vi "WHD_VEten_.WS_BIDIR_Cal_26_01_2024.vi"() -> ()   [LabVIEW 2015]
uses:
  <vilib>/LabVIEW Targets/FPGA/cRIO/shared/nicrio_ModuleControls/nicrio_cRIO-9234_DataRatesRing2.ctl
  <vilib>/RTwatchdog.llb/Watchdog expiration actions.ctl
  <vilib>/userdefined/High Color/nirio_resource_hc.ctl
  <vilib>/Platform/TimedLoop/XDataNode/timing_clust.ctl
  <vilib>/Platform/TimedLoop/XDataNode/nitl_modes.ctl
  <vilib>/Platform/TimedLoop/XDataNode/wakeup.ctl
  <vilib>/Analysis/5stat.llb/RMS (DBL).vi
  <vilib>/FPGAPlugInAG/cRIO-9031/niLvFpga_Open_cRIO-9031.vi
  <vilib>/Utility/error.llb/Error Cluster From Error Code.vi
  <vilib>/rvi/errors/niLvFpgaAdjustHostInterfaceError.vi
  <vilib>/FPGAPlugInAG/cRIO-9031/niLvFpga_Run_cRIO-9031.vi
  <vilib>/rvi/interface/common/niFpgaWaitOnOcc.vi
  <vilib>/Utility/file.llb/Write Delimited Spreadsheet (string).vi
  <vilib>/FPGAPlugInAG/cRIO-9031/niLvFpga_Reset_cRIO-9031.vi
  <vilib>/measure/madcrms.llb/Basic Averaged DC-RMS for 1 Chan.vi
  <vilib>/measure/maspectr.llb/FFT Spectrum (Mag-Phase) for 1 Chan.vi
  <vilib>/Utility/config.llb/Write Key (Double).vi
  <vilib>/FPGAPlugInAG/cRIO-9031/niLvFpga_Close_cRIO-9031.vi
  <vilib>/rvi/interface/nirviOpenFPGA/nirviOpenFPGA.xnode
  FPGA Bitfiles/WRDArabia_FPGATarget_FPGA8a2wsBIdirec_pdg683fU6LY.lvbitx
  <vilib>/rvi/interface/nirviReadWriteControl/nirviReadWriteControl.xnode
  <vilib>/rvi/interface/nirviMethod/nirviMethod.xnode
  <vilib>/platform/TimedLoop/XDataNode/XDataNode.xnode
  <vilib>/rvi/interface/nirviCloseFPGA/nirviCloseFPGA.xnode
  <vilib>/rvi/errors/niLvFpgaMergeErrorWithErrorCode.vi
  AURA_Wheel/Json2Labv.lvlib
  AURA_Wheel/AuraWheelAPI/AuraWheel.lvlib
  NiFpgaLv.dll
  <vilib>/FPGAPlugInAG/cRIO-9031/niLvFpga_ConfigureFifo_cRIO-9031.vi
  <vilib>/FPGAPlugInAG/cRIO-9031/niLvFpga_StartFifo_cRIO-9031.vi
  <vilib>/FPGAPlugInAG/cRIO-9031/niLvFpga_ReadFifo_cRIO-9031.vi
  <vilib>/FPGAPlugInAG/cRIO-9031/niLvFpga_StopFifo_cRIO-9031.vi
  <vilib>/measure/NI_MAPro.lvlib
  <vilib>/Analysis/NI_AALPro.lvlib
  <vilib>/Analysis/NI_AALBase.lvlib
  <vilib>/Utility/config.llb/NI_LVConfig.lvlib
  <vilib>/Platform/TimedLoop/XDataNode/XDNodeRunTimeDep.lvlib
  Library/IF2_Reader/IF2_Reader.lvlib
panel:
  out "Power Status":bool
  out "Diagnostic data":sgl[](array[numeric])
  out "Last Train passes - RFIDs":T1
  out "I2":sgl[](array[numeric])
  out "I1":sgl[](array[numeric])
  out "A8":sgl[](array[numeric])
  out "A7":sgl[](array[numeric])
  out "A6":sgl[](array[numeric])
  out "A5":sgl[](array[numeric])
  out "A4":sgl[](array[numeric])
  out "A3":sgl[](array[numeric])
  out "A2":sgl[](array[numeric])
  out "A1":sgl[](array[numeric])
  out "Accelerometer 8":bool
  out "Accelerometer 7":bool
  out "Accelerometer 6":bool
  out "Accelerometer 5":bool
  out "Accelerometer 4":bool
  out "Accelerometer 3":bool
  out "Accelerometer 2":bool
  out "Accelerometer 1":bool
  out "Wheel detector 2":bool
  out "Wheel Detector 1":bool
  out "Last time checked":string
  out "RFID connection":bool
  out "Internet connection":bool
  out "Inicio diagnosis":timestamp
  out "RFID_status":path=path "c:/RFID/status.csv"
  in  "Diagnosis":bool
  out "T fuera rango":bool
  out "Frequency":dbl[](array[numeric])
  out "Value to compare":dbl[](array[numeric])
  in  "Developer password":string
  out "Waveform Graph":waveform(sgl)[](graph)
  out "min":dbl[](array[numeric])
  out "max":dbl[](array[numeric])
  out "median":dbl[](array[numeric])
  out "mean":dbl[](array[numeric])
  in  "Accelerometer":i32=1 min=1 max=8
  out "Low cutoff freq":dbl
  out "noise_range":dbl
  out "Numeric":i32
  out "Calibration parameter":dbl
  out "Accel.detected":i32
  out "Mean\nfrequency":dbl format="%0.2f"
  out "Nº meas":i32
  out "Array":i32[](array[numeric])
  out "sorted array":i32[](array[numeric])
  out "Array 3":i32[](array[numeric])
  out "max value":i32
  out "max index(es)":i32
  out "element":i32
  out "size(s) 3":i32
  out "size(s)":i32[](array[numeric])
  out "Valid\nindex":i32[](array[numeric])
  out "Acquiring time":dbl
  out "Inicio pasada 2":timestamp
  out "calibration log":path
  out "date/time string 2":string
  out "Folder":path
  in  "Developer commad":string
  out "Save calibration":bool
  out "Pattern amplitude (g)":dbl=1.02
  out "Pattern frequency (Hz)":dbl=159.2
  out "Report":string
  out "AURA wheel test":bool
  out "LOG.txt":path
  out "Report_AURA":string
  out "error FPGA":errorcluster
  out "error AURA":errorcluster
  out "error manipulacion archivos":errorcluster
  out "Response headers":string
  out "Max RMS Ruedas":dbl[][](array[numeric])
  out "TAGs LR6":string[](array[string])
  out "TAGs HEX":string[](array[string])
  out "Parar":bool
  out "result":bool
  out "TAGs":string[](array[string])
  out "Temperatura (ºC)":dbl
  out "V (m/s)":dbl
  out "Digital?":bool=TRUE
  out "Watchdog config":T2={"reset"=FALSE, "occurrence"=FALSE, "trigger protocol"=enum."active high", "trigger line"=enum."none", "disable watchdog on VI exit"=TRUE}
  out "Tiempo de adquisicion":dbl=10.0
  out "Adquirir":bool
  out "Nº Ruedas 1":i32
  out "NºRuedas 2":i32
  out "Disco Duro Disponible (bytes)":i64
  out "Buffer Overflow":bool
  out "Buffer Underflow":bool
  out "Archivo\nvalido?":bool
  out "Número de ejes detectados":i32
  out "Ejes_convoy":i32
  out "Tiempo de paso (s)":dbl
  out "created path":path
  out "Nombre de archivo":path[](array[path])
  out "LR6 IP address":string="192.168.106.94"
  out "Port LR6":u16=2001
  out "Frecuencia de muestreo (Hz)":dbl=25600.0
  out "Escaneos de la FIFO por canal":u32=5000
  out "Tiempo extra al detector de paso (s)":dbl=1.0
  out "dt RMS":dbl=256.0
  out "Frecuencia de muestreo y módulo CRIO":T3=2 items=["51.200 kS/s (NI 9234)"=1, "25.600 kS/s (NI 9234)"=2, "17.067 kS/s (NI 9234)"=3, "12.800 kS/s (NI 9234)"=4, "10.240 kS/s (NI 9234)"=5, "8.533 kS/s (NI 9234)"=6, "7.314 kS/s (NI 9234)"=7, "6.400 kS/s (NI 9234)"=8, "5.689 kS/s (NI 9234)"=9, "5.120 kS/s (NI 9234)"=10, "4.654 kS/s (NI 9234)"=11, "4.267 kS/s (NI 9234)"=12, "3.938 kS/s (NI 9234)"=13, "3.657 kS/s (NI 9234)"=14, "3.413 kS/s (NI 9234)"=15, "3.200 kS/s (NI 9234)"=16, "3.012 kS/s (NI 9234)"=17, "2.845 kS/s (NI 9234)"=18, "2.695 kS/s (NI 9234)"=19, "2.560 kS/s (NI 9234)"=20, "2.438 kS/s (NI 9234)"=21, "2.328 kS/s (NI 9234)"=22, "2.226 kS/s (NI 9234)"=23, "2.133 kS/s (NI 9234)"=24, "2.048 kS/s (NI 9234)"=25, "1.969 kS/s (NI 9234)"=26, "1.896 kS/s (NI 9234)"=27, "1.829 kS/s (NI 9234)"=28, "1.765 kS/s (NI 9234)"=29, "1.707 kS/s (NI 9234)"=30, "1.652 kS/s (NI 9234)"=31]
  out "Puerto RFID":u16=2189
  out "IP RFID":string="192.168.106.99"
  out "Offset_rueda WS 2":fxp<+/-,24,-4>=0.004999998956918716 format="%.27g"
  out "Count(mSec)":u32=2
  out "RFID NEM on?":bool
  out "RFID LR6 on?":bool
  out "Canal cero WS1?":bool
  out "Canal cero WS2":bool
  in  "Calibration":bool
  out "Direccion 0?":bool
  out "Boton Adquirir?":bool
  out "RuedaDetectada2?":bool=TRUE
  out "RuedaDetectada1?":bool=TRUE
  out "Timeout ruedas":dbl
  out "Borrar archivos\nadquisicion con error":bool
  out "Able watchdog?":bool
  out "Reset watchdog?":bool
  out "Leer config RFID NEM":bool
  out "bytes to read":i32
  out "DeviceAddress":u8
  out "timeout ms (60000)":i32
  out "Max archivos":u32=2
  out "Bytes libre despues de borrar":u32=2
  out "Bytes min libre":u32=2
  out "Nº de acelerómetros":i32
  out "Nº inductivos":i32
  out "Offset_rueda WS 1":fxp<+/-,24,-4>=0.004999998956918716 format="%.27g"
  out "TAGs_AURAwheel":string[][](array[string])
  out "Plataformas?":bool
  out "Nº Ejes":i32[](array[numeric])
  out "Nº UTs":i32
  out "it-read-LR6":i32[](array[numeric])
  out "it-LR6":i32
  out "RFID_LR6_Error":errorcluster
  out "Series_flota":string[](array[string])
  out "Tabla_flota":string[][](array[string])
  out "Puntos medios de las ventanas":dbl[][](array[numeric])
  out "configuration file path":path=path "c:/Parametros.cfg"
  out "IP synchr":string
  out "data":cluster{"status":string}
  out "confRFID":path=path "c:/RFID/TAGS.csv"
  out "TAGS leidos":path=path "c:/RFID/TAGS.csv"
  out "Use Aura?":bool
  out "Parametros AuraWheel":string[](array[string])
  out "Parámetros acelerómetros":dbl[](array[numeric])
  out "Fin":bool
  out "Contador":i32=1
  out "Path LOG":path=path "c:/TEST"
  out "Fallo fotocelula":bool
  out "Path_Borrar":path=path "c:/Trenes"
  out "Longitud de la unidad":dbl
  out "Aviso no detección":string
  out "Time to Acquire Block (ms)":i32
  out "Distancia de acelerómetros":dbl[](array[numeric])
  out "Block Size":u32
  out "Distancias generales":dbl[](array[numeric])
  out "Reset del controlador":bool
  out "Parar la aplicación":bool
  out "date/time string":string
  out "Timeout ruedas":bool
  out "Tiempo":dbl
  out "Inicio pasada":timestamp
  out "Ultimo TEST":timestamp
  out "DC OK":string
  out "Aviso temperatura":string
  out "connection ID":refnum<k5>
  # "To check the status of the UPS please check the following LEDs physically in the system:"
  # "10. Bar graph showing the current available supply of the UPS (each bar is a 20%)"
  # "12. Red LED: alarm"
  # "13. Yellow LED: battery working mode"
  # "16. Green LED: Power In OK, mains mode"
  # "Calibration - Noise analysis"
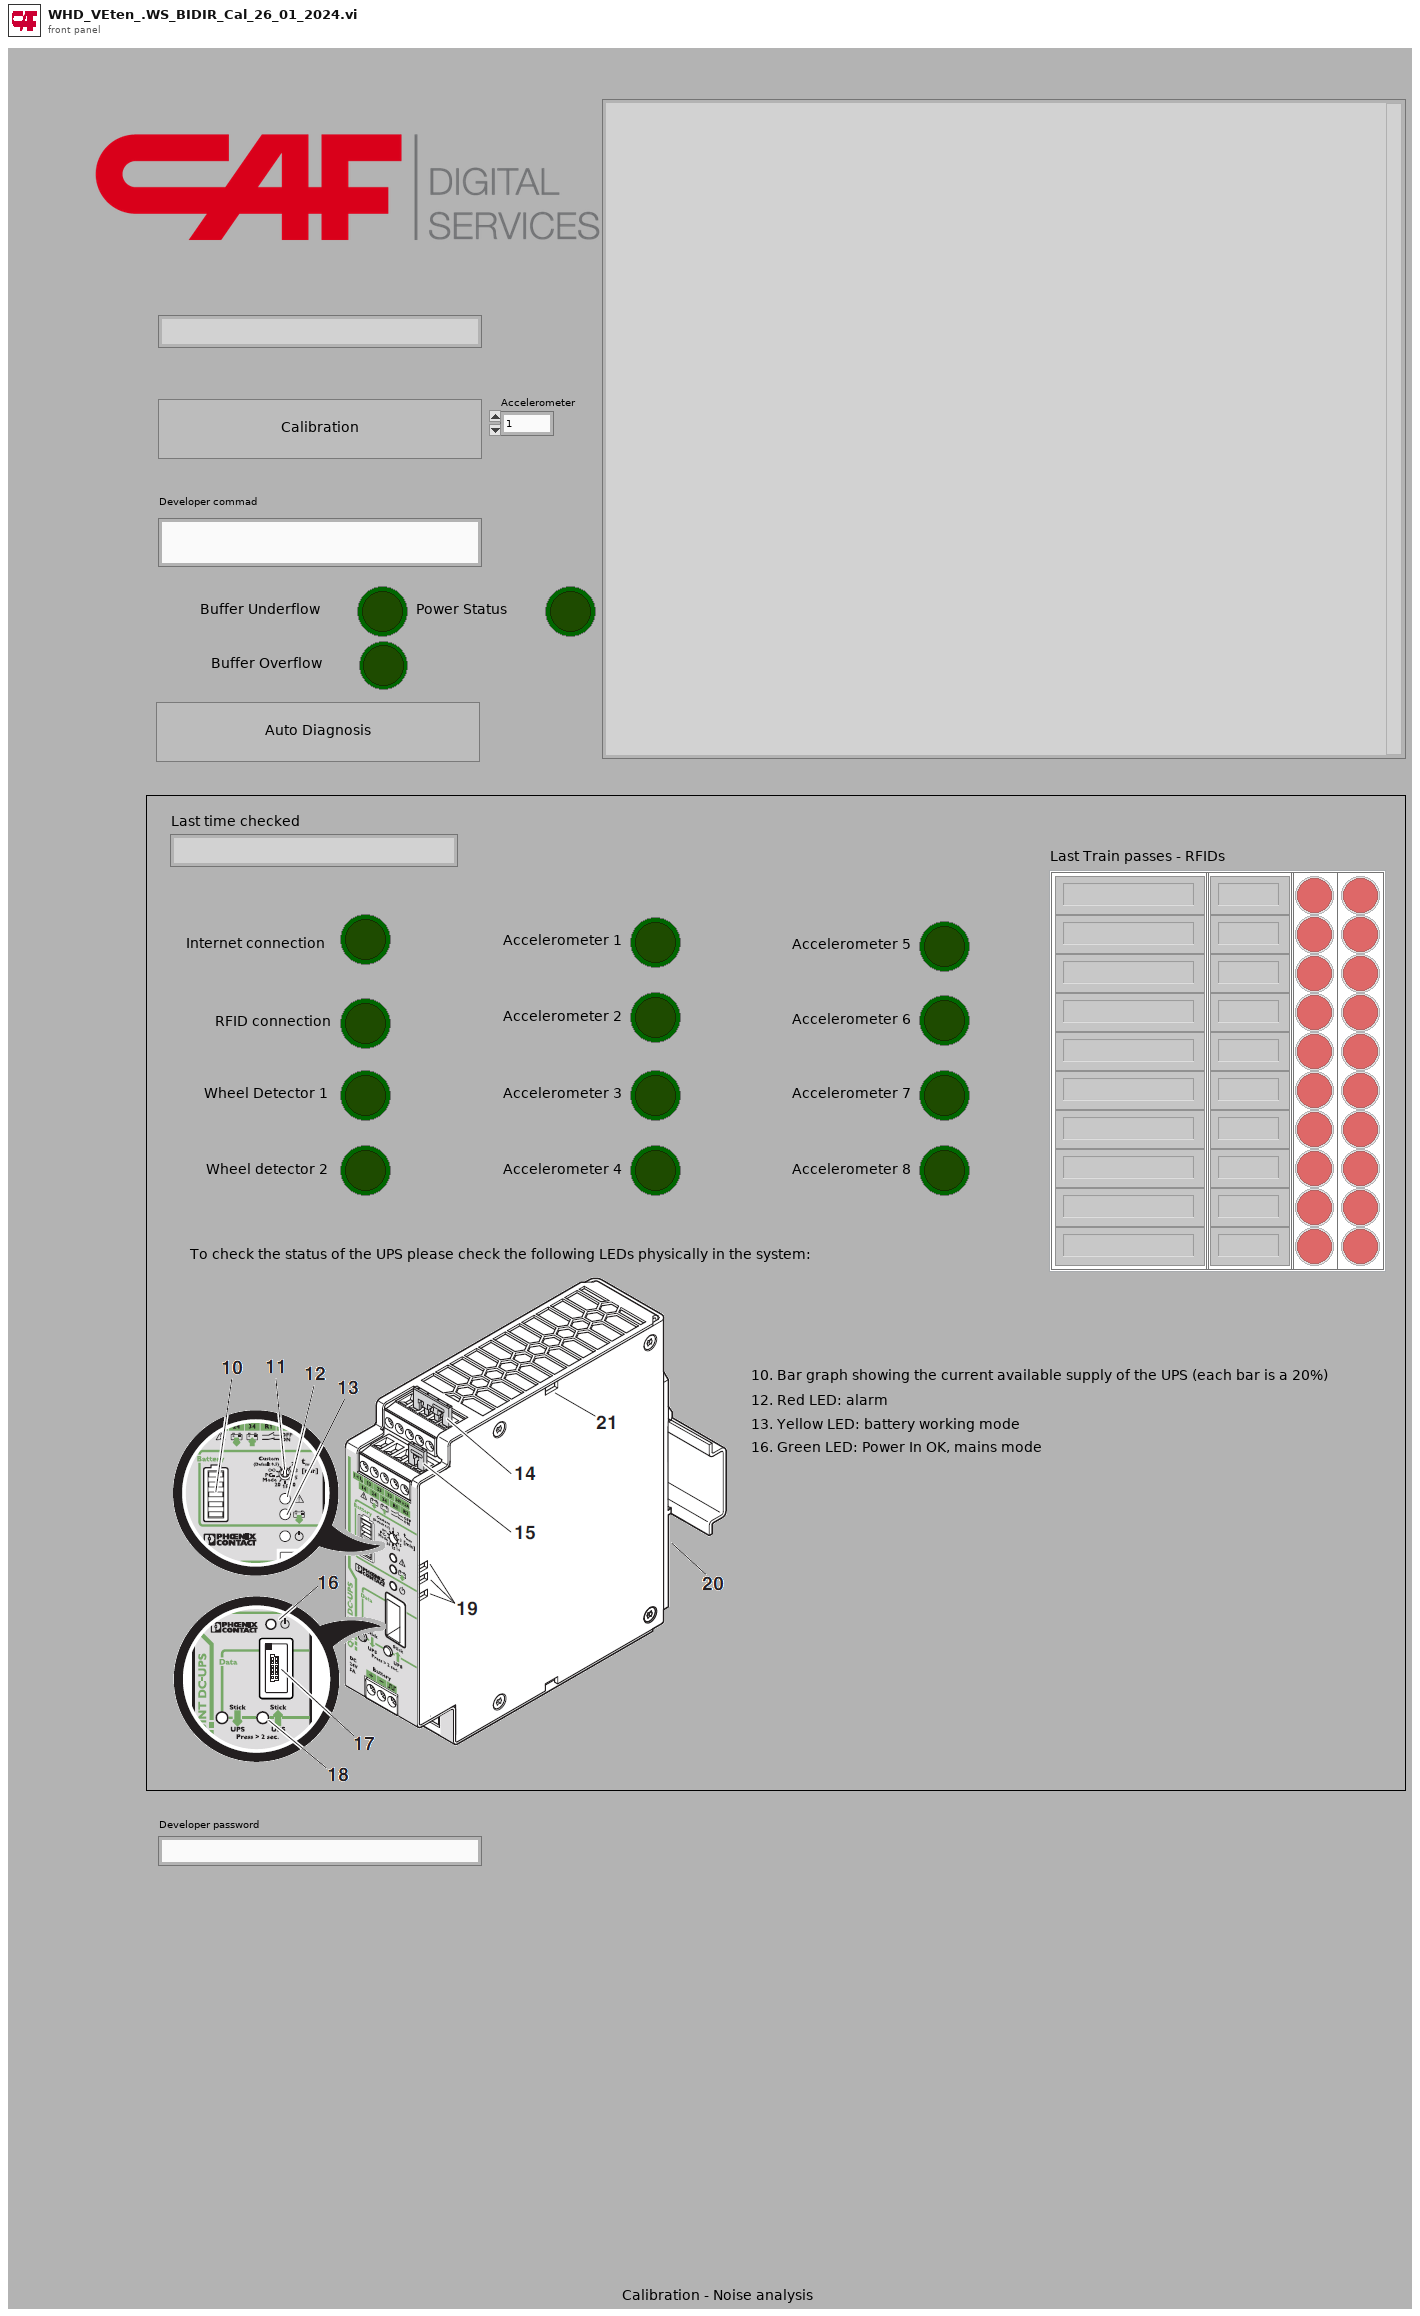
[diagram p1: front panel]
types:
  T1 = cluster{"Array 3":bool[], "Array 4":string[], "Array 6":string[], "Array 5":bool[]}
  T2 = typedef "Watchdog expiration actions.ctl" = cluster{"reset":bool, "occurrence":bool, "trigger protocol":enum16{"active high", "active low", "open collector"}, "trigger line":enum16{"none", "line 0", "line 1", "line 2", "line 3", "line 4", "line 5", "line 6", "line 7", "SMB line 0"}, "disable watchdog on VI exit":bool}
  T3 = typedef "nicrio_cRIO-9234_DataRatesRing2.ctl" = u8
  T4 = typedef "nirio_resource_hc.ctl" = tag
  T5 = enum16{"open", "replace", "create", "open or create", "replace or create", "replace or create with confirmation"}
  T6 = enum16{"big-endian, network order", "native, host order", "little-endian"}
  T7 = typedef "XDNodeRunTimeDep.lvlib/timing_clust.ctl" = cluster{"Expected End [f-1]":u64, "Actual End [f-1]":u64, "Finished Late? [f-1]":bool, "Expected End [i-1]":u64, "Actual End [i-1]":u64, "Finished Late? [i-1]":bool, "Expected Start [i]":u64, "Actual Start [i]":u64, "Expected Start [f]":u64, "Actual Start [f]":u64, "Source Name":string, "Structure Name":string, "Period":i64, "Deadline":i64, "Offset":i64, "Start":i64, "Priority":i32, "Timeout":i32, "Mode":T8, "Wakeup Reason":T9, "Error":errorcluster, "Source Type":string, "Secondary Source Type":string, "Global End Time":u64, "Global Start Time":u64, "Frame Duration":u64, "Iteration Duration":u64, "Assigned CPU":i32, "I/O Scan Engine Mode":u32}
  T8 = typedef "XDNodeRunTimeDep.lvlib/nitl_modes.ctl" = enum32{"No Change", "Process missed periods, maintain original phase", "Discard missed periods, maintain original phase", "Process missed periods, ignore original phase", "Discard missed periods, ignore original phase"}
  T9 = typedef "XDNodeRunTimeDep.lvlib/wakeup.ctl" = enum32{"Normal", "Aborted", "Asynchronous wakeup", "Timing source error", "Timed loop error", "Timeout"}
  T10 = cluster{"error IO":errorcluster, bool[], u32[], string[], dbl[]}
  T11 = cluster{"error out":errorcluster, dbl[], "Normalized Tags":string[], "Direccion 0?":bool}
  T12 = cluster{"g_ts":dbl, "p_sp":dbl, "p_tp":dbl, "p_tg":cluster{"tg_n":dbl, "tg_t":string}[], "p_ax":cluster{"ax_n":dbl, "ax_sp":dbl, "ax_wh":cluster{"wh_p":dbl, "wh_a1":dbl, "wh_a2":dbl, "wh_a3":dbl, "wh_a4":dbl}[]}[]}
  T13 = typedef "NI_LVConfig.lvlib/Config Data RefNum.ctl" = refnum<k1>
  T14 = cluster{"IP":string, "Port":u16, "ReaderConfigFile":path, "ROspecConfigFile":path}
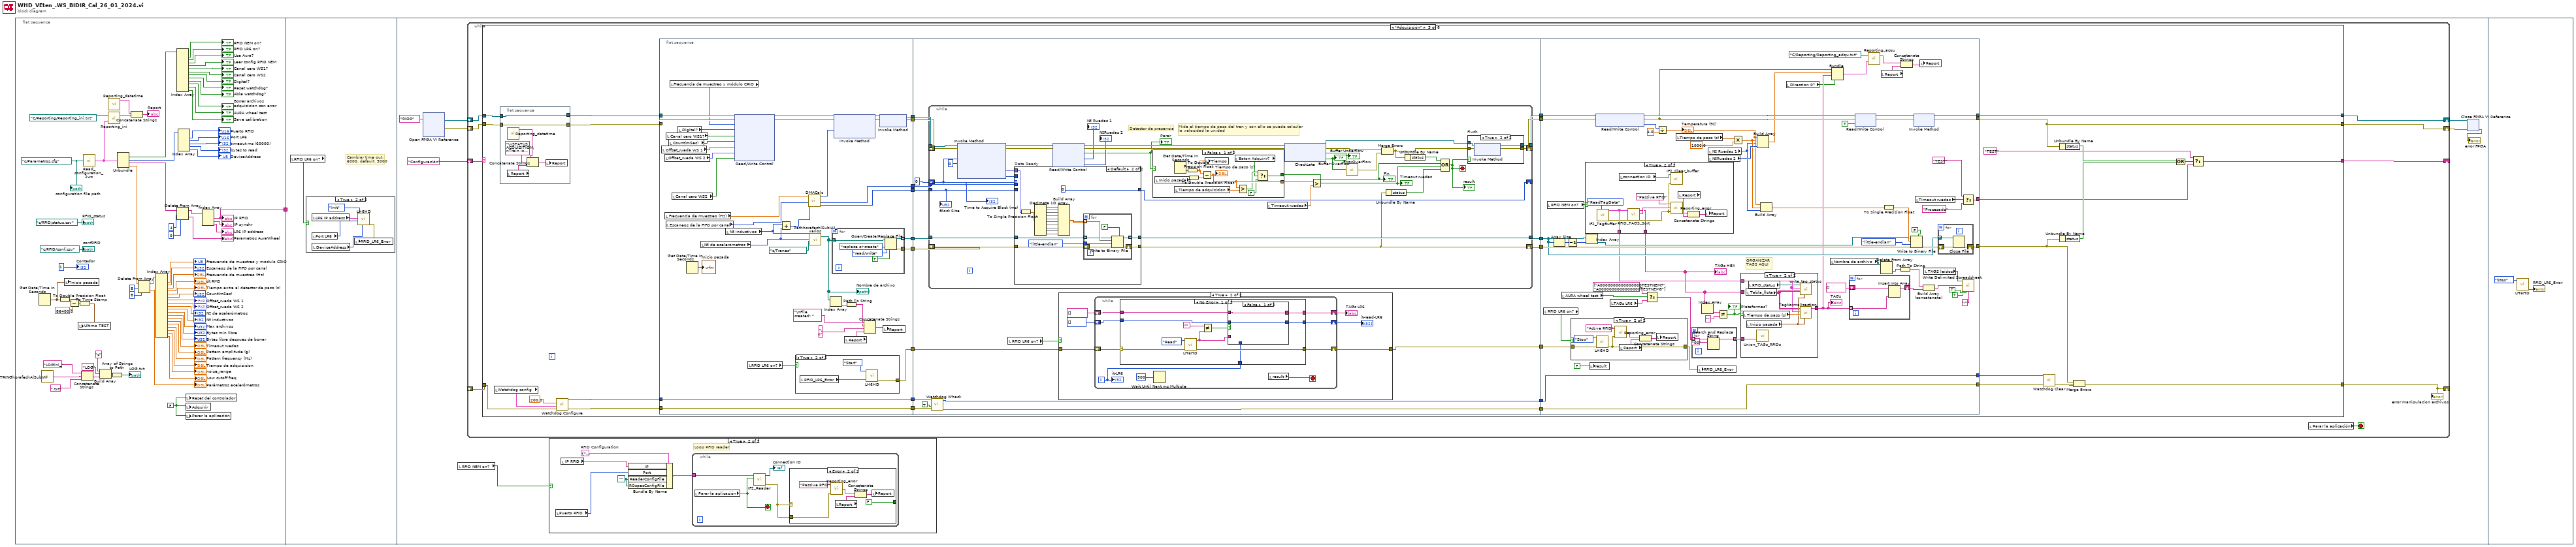
[diagram p0: block diagram]
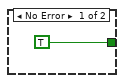
[diagram p4: hidden frame]
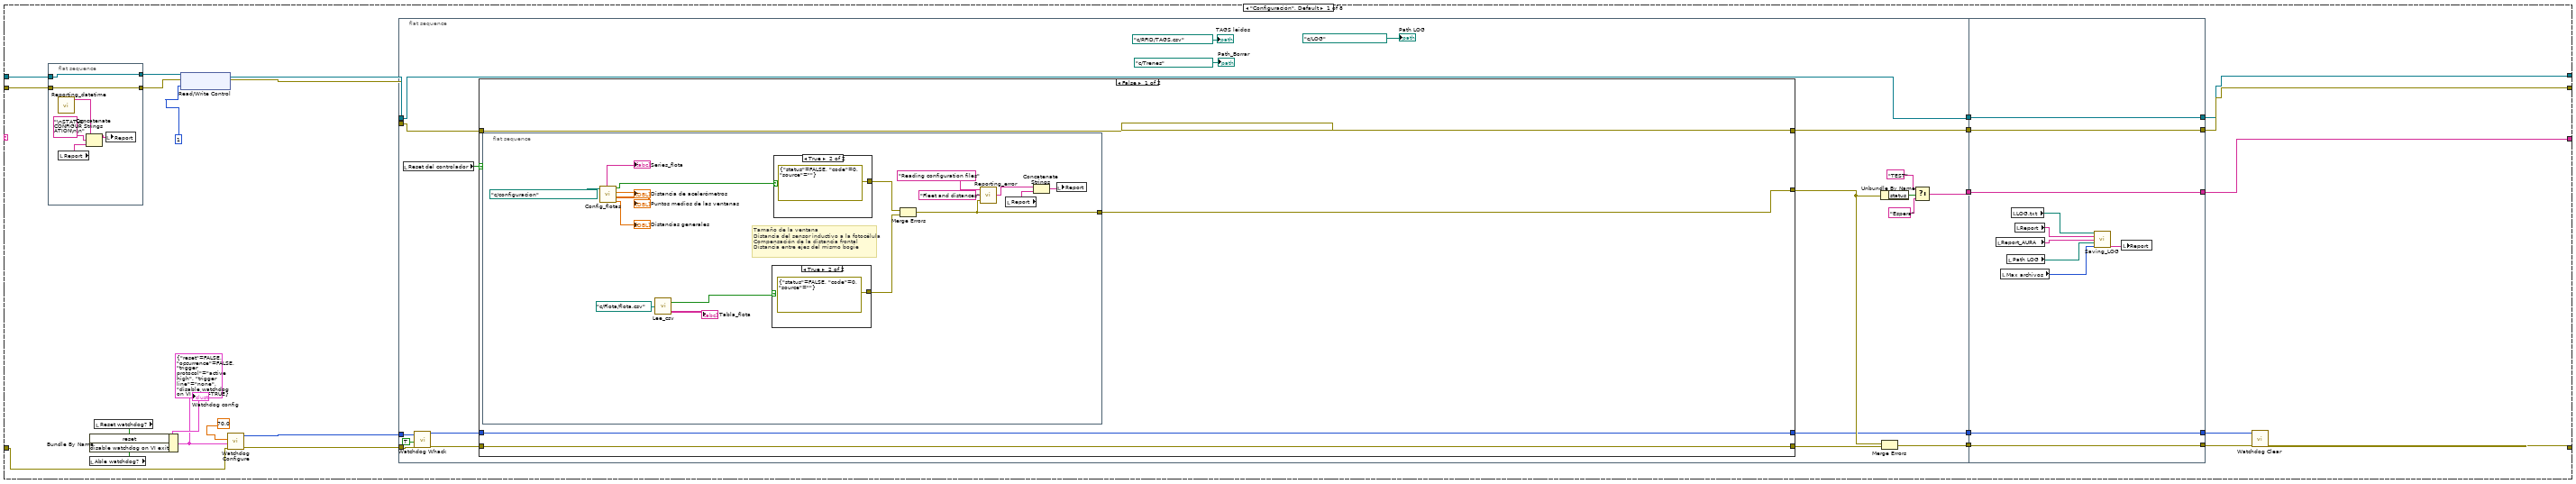
[diagram p5: hidden frame]
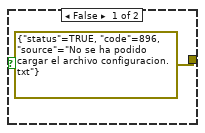
[diagram p6: hidden frame]
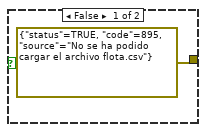
[diagram p7: hidden frame]
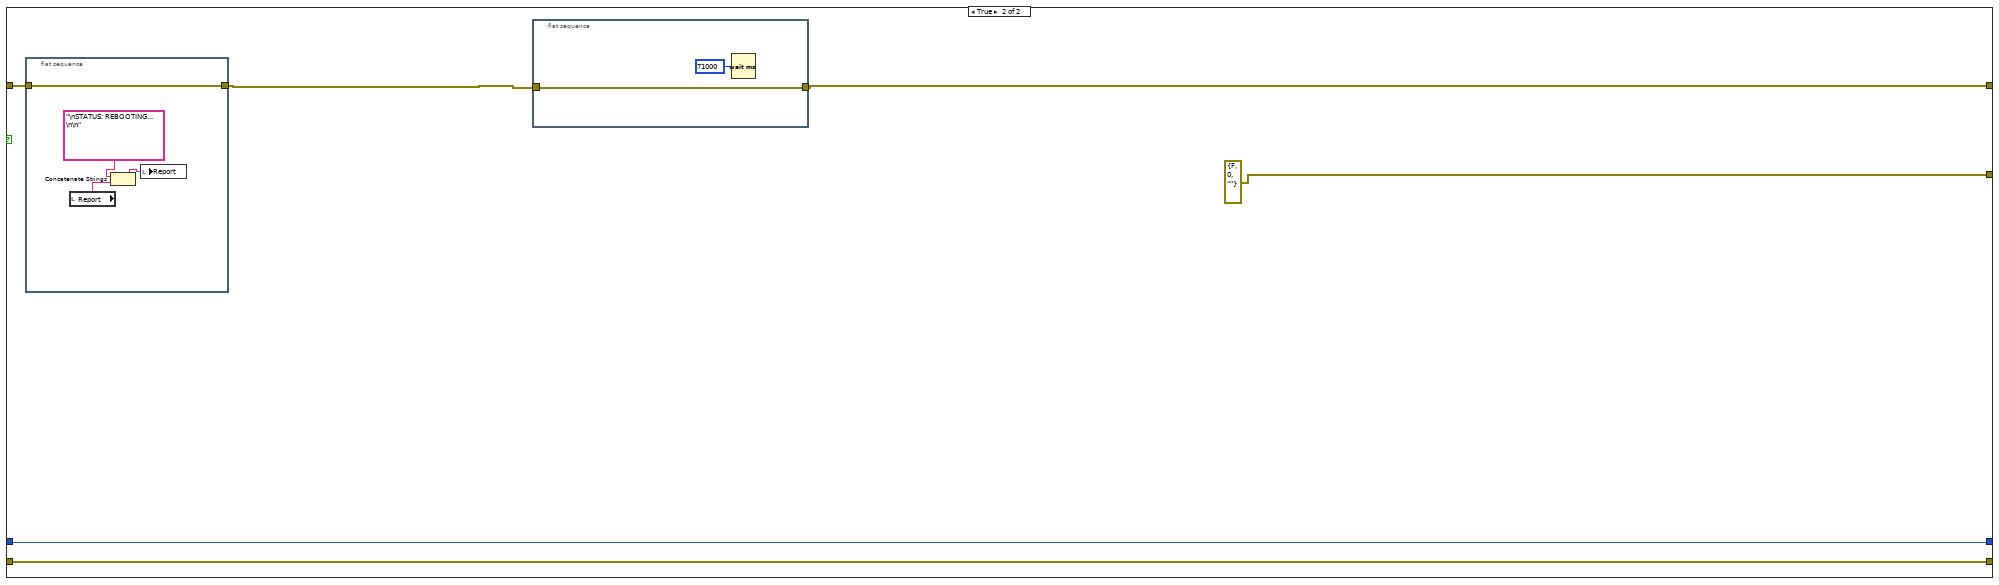
[diagram p8: hidden frame]
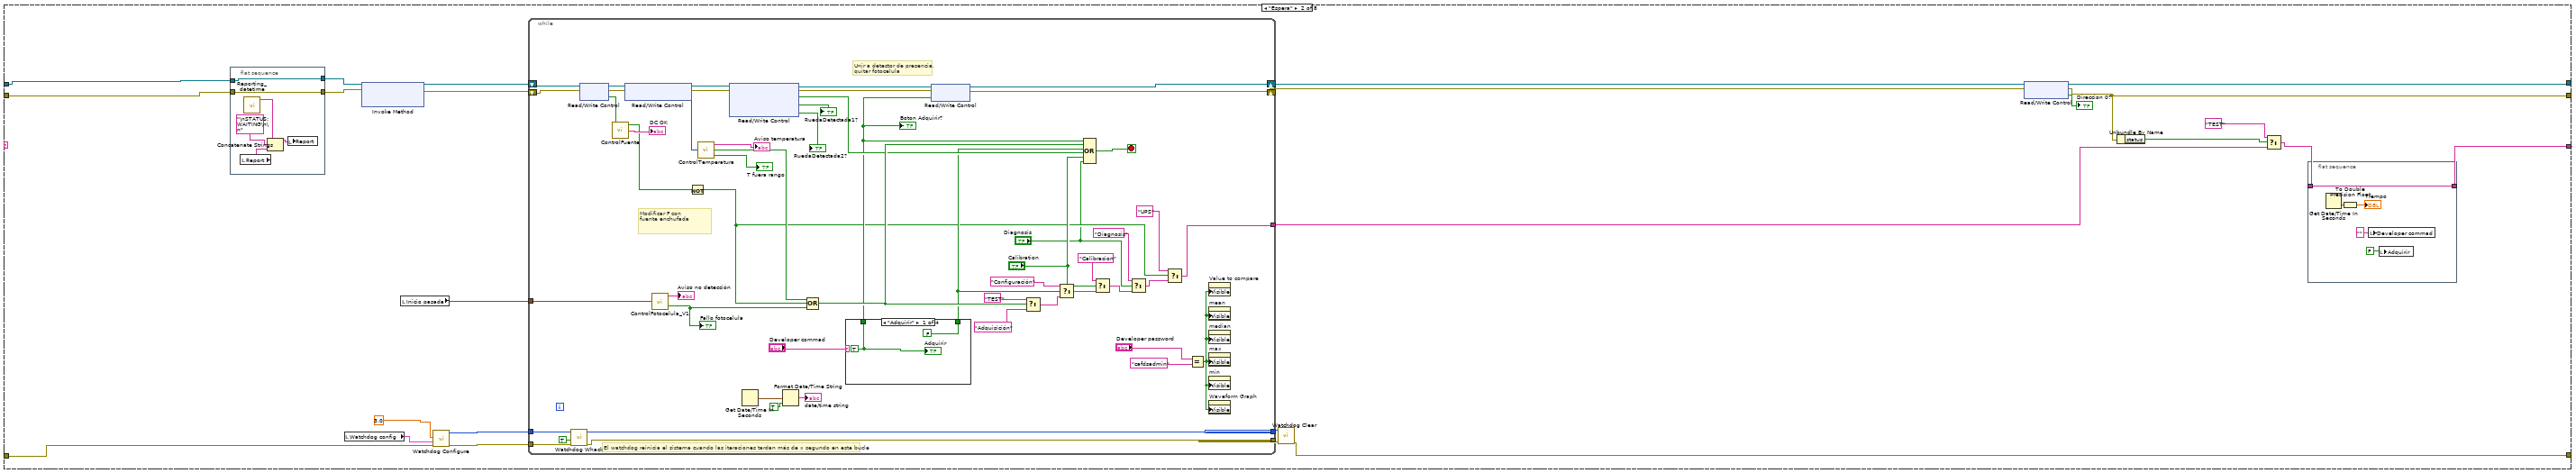
[diagram p9: hidden frame]
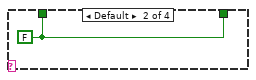
[diagram p10: hidden frame]
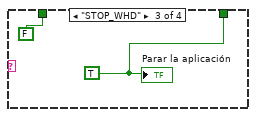
[diagram p11: hidden frame]
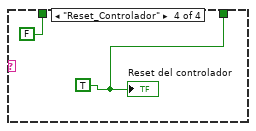
[diagram p12: hidden frame]
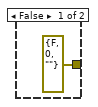
[diagram p13: hidden frame]
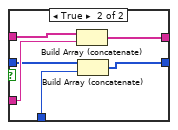
[diagram p15: hidden frame]
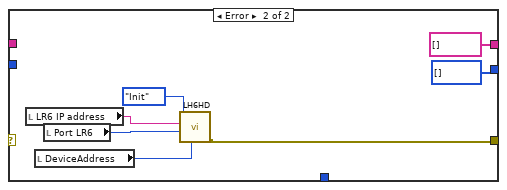
[diagram p16: hidden frame]
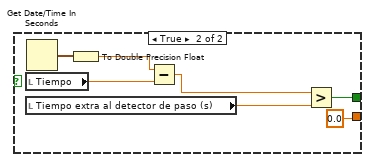
[diagram p17: hidden frame]
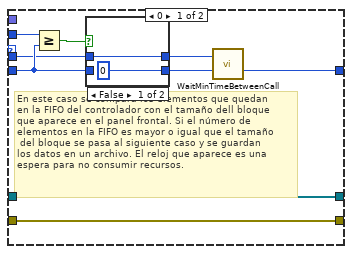
[diagram p18: hidden frame]
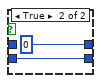
[diagram p19: hidden frame]
diagram:
  n1 = flat-sequence {
    tunnel: [w5] -> w1
    tunnel: w1 -> [_]
    frame #0 {
      w6 = FALSE ("Reset del controlador")
      w67 = path "c:/Parametros.cfg" ("configuration file path")
      n2 = Get Date/Time In Seconds() -> (seconds since 1Jan1904=w72:timestamp)
      n3 = call "STRINGhorafechA(SubVI).vi"() -> ("STRINGhora_fecha"=w17:string)
      n4 = To Double Precision Float(number=w72) -> (double precision float=w74:dbl)
      n5 = local write "Inicio pasada"(w72) -> ()
      n6 = Subtract(x=w74, y=86400.0) -> (x-y=w73:dbl)
      n7 = To Time Stamp(1:w73) -> (0:w71:timestamp)
      n8 = local write "Ultimo TEST"(w71) -> ()
      n9 = Concatenate Strings("LOGini_" ("string"), w17, ".txt" ("string")) -> (w19:string)
      n10 = call "Read_configuration_2ws.vi"("configuration file path"=w67) -> ("output cluster"=w23:T10)
      n11 = Build Array("c", "LOG" ("element"), w19) -> (w16:string[])
      n12 = call "Reporting_ini.vi"("Configuration cluster"=w23, "address repoting"=path "C:/Reporting/Reporting_ini.txt" ("file (use dialog)")) -> ("Reporting"=w22:string)  [unwired: 1 in]
      n13 = call "Reporting_datetime.vi"() -> ("String"=w20:string)  [unwired: 11 in]
      n14 = Array of Strings to Path(0:w16) -> (2:→"LOG.txt":path)  [unwired: 1 out]
      n15 = Unbundle(w23) -> (w70:bool[], w69:u32[], w62:string[], w66:dbl[])  [unwired: 1 out]
      n16 = Concatenate Strings(w20, w22) -> (→"Report":string)
      n17 = Delete From Array(array=w66, length=8, index=8) -> (deleted portion=→"Parámetros acelerómetros":dbl[], array with subset deleted=w65:dbl[])
      n18 = Index Array(array=w65) -> (element #1=→"Frecuencia de muestreo y módulo CRIO":dbl, element #2=→"Escaneos de la FIFO por canal":dbl, element #3=→"Frecuencia de muestreo (Hz)":dbl, element #4=→"dt RMS":dbl, element #5=→"Tiempo extra al detector de paso (s)":dbl, element #6=→"Count(mSec)":dbl, element #7=→"Offset_rueda WS 1":dbl, element #8=→"Offset_rueda WS 2":dbl, element #9=→"Nº de acelerómetros":dbl, element #10=→"Nº inductivos":dbl, element #11=→"Max archivos":dbl, element #12=→"Bytes min libre":dbl, element #13=→"Bytes libre despues de borrar":dbl, element #14=→"Timeout ruedas":dbl, element #15=→"Pattern amplitude (g)":dbl, element #16=→"Pattern frequency (Hz)":dbl, element #17=→"Tiempo de adquisicion":dbl, element #18=→"noise_range":dbl, element #19=→"Low cutoff freq":dbl)  [unwired: 19 in]
      n19 = Index Array(array=w70) -> (element #1=→"RFID NEM on?":bool, element #2=→"RFID LR6 on?":bool, element #3=→"Use Aura?":bool, element #4=→"Leer config RFID NEM":bool, element #5=→"Canal cero WS1?":bool, element #6=→"Canal cero WS2":bool, element #7=→"Digital?":bool, element #8=→"Reset watchdog?":bool, element #9=→"Able watchdog?":bool, element #10=→"Borrar archivos\nadquisicion con error":bool, element #11=→"AURA wheel test":bool, element #12=→"Save calibration":bool)  [unwired: 12 in]
      n20 = Delete From Array(array=w62, length=4, index=0) -> (deleted portion=→"Parametros AuraWheel":string[], array with subset deleted=w61:string[])
      n21 = Index Array(array=w69) -> (element #1=→"Puerto RFID":u32, element #2=→"Port LR6":u32, element #3=→"timeout ms (60000)":u32, element #4=→"bytes to read":u32, element #5=→"DeviceAddress":u32)  [unwired: 5 in]
      n22 = local write "Reset del controlador"(w6) -> ()
      n23 = local write "Adquirir"(w6) -> ()
      n24 = local write "Parar la aplicación"(w6) -> ()
      n25 = Index Array(array=w61) -> (element #1=w5:string, element #2=→"IP synchr":string, element #3=→"LR6 IP address":string)  [unwired: 3 in]
      "IP RFID" <- w5
      "Contador" <- 1
      "confRFID" <- path "c:/RFID/conf.csv" ("file path (use dialog)")
      "configuration file path" <- w67
      "RFID_status" <- path "c:/RFID/status.csv" ("file path (use dialog)")
    }
    frame #1 {
      # "Cambiar time out:\n6000, default, 5000"
      n26 = local read "RFID LR6 on?"() -> (w76:bool)
      n27 = case shown="True" w76 {
        frame False {
        }
        frame True {
          n28 = local read "LR6 IP address"() -> (w77:string)
          n29 = local read "Port LR6"() -> (w78:u16)
          n30 = local read "DeviceAddress"() -> (w79:u8)
          n31 = call "LH6HD.vi"("DeviceAddress"=w79, "Reader Port"=w78, "IP Address"=w77, "Action"=enum16{"Init", "Start", "Read", "Stop", "Exit"}."Init") -> ("error out"=w81:errorcluster)  [unwired: 6 in, 1 out]
          n32 = local write "RFID_LR6_Error"(w81) -> ()
        }
      }
    }
    frame #2 {
      n33 = xnode "Open FPGA VI Reference"("resource name"=T4 "RIO0") -> ("FPGA VI Reference Out"=w89:refnum<k20>, "error out"=w88:errorcluster)  [unwired: 1 in]
      n34 = local read "RFID NEM on?"() -> (w82:bool)
      n35 = while {
        shift-right: [w107] -> _
        shift-left: "Configuración" -> [w114]
        shift-right: [w106] -> w85
        shift-left: w89 -> [w113]
        shift-right: [w108] -> w84
        shift-left: w88 -> [w112]
        shift-right: [w111] -> _
        shift-left: _ -> [w110]
        stop <- w109 stop-if-true
        n36 = case shown="\"Adquisición\"" w114 {
          tunnel: [w129 w232 w328 w679 w927 "Espera" "Espera" ("t") "Espera" ("t")] -> w107
          tunnel: [w139 w221 w342 w668 w926 w995 w1796 w1818] -> w106
          tunnel: [w140 w220 w343 w666 w925 w993 w1795 w1827] -> w108
          tunnel: w113 -> [w123 w219 w314 w669 w926 w1005 w1797 w1836]
          tunnel: w112 -> [w122 w218 w313 w667 w918 w1004 w1792 w1838]
          tunnel: [w136 w226 w340 w664 w917 w994 w1793 w1819] -> w111
          tunnel: w110 -> [w128 w231 w324 w678 w914 w994 w1793 w1819]
          frame "Configuración", Default {
            n37 = flat-sequence {
              tunnel: w123 -> [w146]
              tunnel: w122 -> [w145]
              tunnel: [w146] -> w121
              tunnel: [w145] -> w120
              frame #0 {
                n38 = call "Reporting_datetime.vi"() -> ("String"=w141:string)  [unwired: 11 in]
                n39 = local read "Report"() -> (w142:string)
                n40 = Concatenate Strings(w141, "\nSTATUS: CONFIGURATION\n\n", w142) -> (w144:string)
                n41 = local write "Report"(w144) -> ()
              }
            }
            n42 = local read "Able watchdog?"() -> (w133:bool)
            n43 = local read "Reset watchdog?"() -> (w134:bool)
            n44 = Bundle By Name(cluster=T2 {"reset"=FALSE, "occurrence"=FALSE, "trigger protocol"=enum."active high", "trigger line"=enum."none", "disable watchdog on VI exit"=TRUE} ("expiration actions"), "reset"=w134, "disable watchdog on VI exit"=w133) -> (w127:T2)
            "Watchdog config" <- w127
            n45 = xnode "Read/Write Control"("FPGA VI Reference In"=w121, "error in"=w120, "Cycles to Filter"=u16 1) -> ("FPGA VI Reference Out"=w132:refnum<k20>, "error out"=w131:errorcluster)
            n46 = call <vilib>:"Watchdog Configure.vi"("error in (no error)"=w128, "expiration actions"=w127, "timeout (1 sec)"=70.0) -> ("error out"=w124:errorcluster, "watchdogID"=w125:u64)  [unwired: 1 in, 2 out]
            n47 = flat-sequence {
              tunnel: w132 -> [w158]
              tunnel: w131 -> [w155]
              tunnel: w125 -> [w148]
              tunnel: w124 -> [w147]
              tunnel: [w157] -> w119
              tunnel: [w165] -> w118
              tunnel: [w158] -> w117
              tunnel: [w160] -> w116
              tunnel: [w152] -> w115
              tunnel: [w210] -> w138
              tunnel: [w211] -> w137
              tunnel: [w212] -> w139
              tunnel: [w213] -> w129
              tunnel: [w214] -> w140
              tunnel: w119 -> [w214]
              tunnel: w118 -> [w213]
              tunnel: w117 -> [w212]
              tunnel: w116 -> [w211]
              tunnel: w115 -> [w210]
              frame #0 {
                n48 = local read "Reset del controlador"() -> (w154:bool)
                n49 = call <vilib>:"Watchdog Whack.vi"("error in (no error)"=w147, "reset watchdog after expire? (F)"=TRUE, "watchdogID in"=w148) -> ("error out"=w150:errorcluster, "watchdogID out"=w151:u64)  [unwired: 2 in, 1 out]
                n50 = case shown="False" w154 {
                  tunnel: w155 -> [w170 w193]
                  tunnel: [w170 w196] -> w157
                  tunnel: [w167 errorcluster {"status"=FALSE, "code"=0, "source"=""} ("error IO")] -> w156
                  tunnel: [w169 w195] -> w152
                  tunnel: w151 -> [w169 w195]
                  tunnel: w150 -> [w168 w194]
                  tunnel: [w168 w194] -> w149
                  frame False {
                    n51 = flat-sequence {
                      tunnel: [w171] -> w167
                      frame #0 {
                        # "Tamaño de la ventana\nDistancia del sensor inductivo a la fotocélula\nCompensación de la distancia frontal\nDistancia entre ejes del mismo bogie"
                        n52 = call "Config_flotas.vi"("file path (dialog if empty)"=path "c:/configuracion") -> ("Distancias generales"=→"Distancias generales":dbl[], "Puntos medios de las ventanas"=→"Puntos medios de las ventanas":dbl[][], "Distancia de acelerómetros"=→"Distancia de acelerómetros":dbl[], "Distacias y medidas de dispositivos"=w184:bool, "Series_flota"=→"Series_flota":string[])  [unwired: 3 in]
                        n53 = call "Lee_csv.vi"("Path"=path "c:/Flota/flota.csv") -> ("Tabla_flota"=→"Tabla_flota":string[][], "Lectura_OK?"=w181:bool)
                        n54 = case shown="True" w181 {
                          tunnel: [errorcluster {"status"=TRUE, "code"=895, "source"="No se ha podido cargar el archivo flota.csv"} ("error out") errorcluster {"status"=FALSE, "code"=0, "source"=""} ("error out")] -> w185
                          frame False {
                          }
                          frame True {
                          }
                        }
                        n55 = case shown="True" w184 {
                          tunnel: [errorcluster {"status"=TRUE, "code"=896, "source"="No se ha podido cargar el archivo configuracion.txt"} ("error out") errorcluster {"status"=FALSE, "code"=0, "source"=""} ("error out")] -> w186
                          frame False {
                          }
                          frame True {
                          }
                        }
                        n56 = Merge Errors(w186, w185) -> (w171:errorcluster)
                        n57 = call "Reporting_error.vi"("error out 2"=w171, "Concept explanation"="Fleet and distances", "Concept"="Reading configuration files") -> ("Reporting"=w173:string)
                        n58 = local read "Report"() -> (w172:string)
                        n59 = Concatenate Strings(w173, w172) -> (w174:string)
                        n60 = local write "Report"(w174) -> ()
                      }
                    }
                  }
                  frame True {
                    n61 = flat-sequence {
                      tunnel: w193 -> [w201]
                      tunnel: [w201] -> w192
                      frame #0 {
                        n62 = local read "Report"() -> (w200:string)
                        n63 = Concatenate Strings("\nSTATUS: REBOOTING...\n\n", w200) -> (w198:string)
                        n64 = local write "Report"(w198) -> ()
                      }
                    }
                    n65 = flat-sequence {
                      tunnel: [w203] -> w196
                      tunnel: w192 -> [w203]
                      frame #0 {
                        n66 = Wait (ms)(milliseconds to wait=u32 71000) -> ()  [unwired: 1 out]
                      }
                    }
                  }
                }
                n67 = Unbundle By Name(w156) -> ("status"=w166:bool)
                n68 = Merge Errors(w156, w149) -> (w160:errorcluster)
                n69 = Select(t="TEST", s=w166, f="Espera") -> (s? t:f=w165:string)
                "Path_Borrar" <- path "c:/Trenes" ("file path (use dialog)")
                "Path LOG" <- path "c:/LOG" ("file path (use dialog)")
                "TAGS leidos" <- path "c:/RFID/TAGS.csv" ("file path (use dialog)")
              }
              frame #1 {
                n70 = local read "Report_AURA"() -> (w207:string)
                n71 = local read "Max archivos"() -> (w208:u32)
                n72 = local read "Path LOG"() -> (w209:path)
                n73 = local read "LOG.txt"() -> (w204:path)
                n74 = local read "Report"() -> (w206:string)
                n75 = call "Saving_LOG.vi"("Path"=w204, "Report"=w206, "Report AURA"=w207, "Path Carpeta"=w209, "Nº Archivos Max"=w208) -> ("Report"=w205:string)  [unwired: 9 in, 1 out]
                n76 = local write "Report"(w205) -> ()
              }
            }
            n77 = call <vilib>:"Watchdog Clear.vi"("error in (no error)"=w137, "watchdogID in"=w138) -> ("error out"=w136:errorcluster)  [unwired: 5 in]
          }
          frame "Espera" {
            n78 = flat-sequence {
              tunnel: w219 -> [w245]
              tunnel: w218 -> [w244]
              tunnel: [w245] -> w217
              tunnel: [w244] -> w216
              frame #0 {
                n79 = local read "Report"() -> (w241:string)
                n80 = call "Reporting_datetime.vi"() -> ("String"=w240:string)  [unwired: 11 in]
                n81 = Concatenate Strings(w240, "\nSTATUS: WAITING\n\n", w241) -> (w243:string)
                n82 = local write "Report"(w243) -> ()
              }
            }
            n83 = local read "Watchdog config"() -> (w225:T2)
            n84 = xnode "Invoke Method"("FPGA VI Reference In"=w217, "error in"=w216) -> ("FPGA VI Reference Out"=w235:refnum<k20>, "error out"=w234:errorcluster)  [unwired: 1 in]
            n85 = local read "Inicio pasada"() -> (w239:timestamp)
            n86 = call <vilib>:"Watchdog Configure.vi"("error in (no error)"=w231, "expiration actions"=w225, "timeout (1 sec)"=3.0) -> ("error out"=w230:errorcluster, "watchdogID"=w229:u64)  [unwired: 1 in, 2 out]
            n87 = while {
              tunnel: [w260] -> w238
              shift-right: [w275] -> w222
              shift-left: w235 -> [w283]
              shift-right: [w274] -> w215
              shift-left: w234 -> [w282]
              tunnel: w239 -> [w286]
              tunnel: w230 -> [w272]
              tunnel: w229 -> [w273]
              tunnel: [w271] -> w228
              tunnel: [w270] -> w227
              stop <- w265 stop-if-true
              # "Modificar F con\nfuente enchufada"
              # "Unir a detector de presencia,\nquitar fotocelula"
              # "El watchdog reinicia el sistema cuando las iteraciones tardan más de x segundo en este bucle"
              n88 = call <vilib>:"Watchdog Whack.vi"("error in (no error)"=w272, "reset watchdog after expire? (F)"=TRUE, "watchdogID in"=w273) -> ("error out"=w270:errorcluster, "watchdogID out"=w271:u64)  [unwired: 2 in, 1 out]
              n89 = xnode "Read/Write Control"("FPGA VI Reference In"=w283, "error in"=w282) -> ("FPGA VI Reference Out"=w295:refnum<k20>, "error out"=w294:errorcluster, "DC OK"=w299:bool)
              n90 = call "ControlFuente.vi"("DC OK 3"=w299) -> ("DC OK 2"=w261:bool, "DC OK"=→"DC OK":string)  [unwired: 1 out]
              n91 = xnode "Read/Write Control"("FPGA VI Reference In"=w295, "error in"=w294) -> ("FPGA VI Reference Out"=w290:refnum<k20>, "error out"=w289:errorcluster, "Chassis Temperature"=w297:i16)
              n92 = call "ControlFotocelula_V1.vi"("Tiempo de entrada a espera"=w286) -> ("Aviso no detección"=→"Aviso no detección":string, "Boolean"=w287:bool)
              "Fallo fotocelula" <- w287
              n93 = Not(x=w261) -> (.not. x?=w259:bool)
              n94 = call "ControlTemperatura.vi"("Chassis Temperature"=w297) -> ("Aviso temperatura"=→"Aviso temperatura":string, "Boolean"=w291:bool, "T fuera rango"=→"T fuera rango":bool)
              n95 = xnode "Read/Write Control"("FPGA VI Reference In"=w290, "error in"=w289) -> ("FPGA VI Reference Out"=w285:refnum<k20>, "error out"=w284:errorcluster, "Detector de presencia"=w278:bool, "RuedaDetectada1?"=→"RuedaDetectada1?":bool, "RuedaDetectada2?"=→"RuedaDetectada2?":bool)
              n96 = Get Date/Time In Seconds() -> (seconds since 1Jan1904=w280:timestamp)
              n97 = Format Date/Time String(seconds (now)=w280, UTC format=TRUE) -> (date/time string=→"date/time string":string)  [unwired: 1 in]
              n98 = Compound Arithmetic op=OR(w291, w259, w287) -> (w288:bool)
              n99 = case shown="\"Adquirir\"" "Developer commad" {
                tunnel: [w305 w306 FALSE ("Adquirir") FALSE ("Adquirir")] -> w264
                tunnel: [FALSE ("Adquirir") w306 w307 w309] -> w263
                frame "Adquirir" {
                  w305 = TRUE ("Adquirir")
                  "Adquirir" <- w305
                }
                frame Default {
                  w306 = FALSE ("Adquirir")
                }
                frame "STOP_WHD" {
                  w307 = TRUE ("Adquirir")
                  "Parar la aplicación" <- w307
                }
                frame "Reset_Controlador" {
                  w309 = TRUE ("Adquirir")
                  "Reset del controlador" <- w309
                }
              }
              "Boton Adquirir?" <- w264
              n100 = xnode "Read/Write Control"("FPGA VI Reference In"=w285, "error in"=w284, "Fotocélula"=w264) -> ("FPGA VI Reference Out"=w275:refnum<k20>, "error out"=w274:errorcluster)
              n101 = Select(t="TEST", s=w288, f="Adquisición") -> (s? t:f=w300:string)
              n102 = Select(t="Configuración", s=w263, f=w300) -> (s? t:f=w268:string)
              n103 = Compound Arithmetic op=OR(w264, w288, w263, w278, "Calibration", "Diagnosis") -> (w265:bool)
              n104 = Select(t="Calibracion", s="Calibration", f=w268) -> (s? t:f=w254:string)
              n105 = Select(t="Diagnosis", s="Diagnosis", f=w254) -> (s? t:f=w252:string)
              n106 = Select(t="UPS", s=w259, f=w252) -> (s? t:f=w260:string)
              n107 = Equal?(x="Developer password", y="cafdsadmin") -> (x = y?=w256:bool)
              n108 = property on="Value to compare" class="Arr (strict)"("Visible"=w256) -> ()  [unwired: 2 in, 2 out]
              n109 = property on="mean" class="Arr (strict)"("Visible"=w256) -> ()  [unwired: 2 in, 2 out]
              n110 = property on="median" class="Arr (strict)"("Visible"=w256) -> ()  [unwired: 2 in, 2 out]
              n111 = property on="max" class="Arr (strict)"("Visible"=w256) -> ()  [unwired: 2 in, 2 out]
              n112 = property on="min" class="Arr (strict)"("Visible"=w256) -> ()  [unwired: 2 in, 2 out]
              n113 = property on="Waveform Graph" class="WFGraph (strict)"("Visible"=w256) -> ()  [unwired: 2 in, 2 out]
            }
            n114 = call <vilib>:"Watchdog Clear.vi"("error in (no error)"=w227, "watchdogID in"=w228) -> ("error out"=w226:errorcluster)  [unwired: 5 in]
            n115 = xnode "Read/Write Control"("FPGA VI Reference In"=w222, "error in"=w215) -> ("FPGA VI Reference Out"=w221:refnum<k20>, "error out"=w220:errorcluster, "Direccion 0?"=→"Direccion 0?":bool)
            n116 = Unbundle By Name(w220) -> ("status"=w237:bool)
            n117 = Select(t="TEST", s=w237, f=w238) -> (s? t:f=w233:string)
            n118 = flat-sequence {
              tunnel: [w249] -> w232
              tunnel: w233 -> [w249]
              frame #0 {
                n119 = Get Date/Time In Seconds() -> (seconds since 1Jan1904=w250:timestamp)
                n120 = To Double Precision Float(number=w250) -> (double precision float=→"Tiempo":dbl)
                n121 = local write "Developer commad"("" ("Developer commad")) -> ()
                n122 = local write "Adquirir"(FALSE ("Adquirir")) -> ()
              }
            }
          }
          frame "Adquisición" {
            n123 = local read "Watchdog config"() -> (w325:T2)
            n124 = flat-sequence {
              tunnel: w314 -> [w354]
              tunnel: w313 -> [w353]
              tunnel: [w354] -> w312
              tunnel: [w353] -> w311
              frame #0 {
                n125 = local read "Report"() -> (w350:string)
                n126 = call "Reporting_datetime.vi"() -> ("String"=w349:string)  [unwired: 11 in]
                n127 = Concatenate Strings(w349, "\nSTATUS: ACQUISITION\nTrain is passing\n\n", w350) -> (w352:string)
                n128 = local write "Report"(w352) -> ()
              }
            }
            n129 = call <vilib>:"Watchdog Configure.vi"("error in (no error)"=w324, "expiration actions"=w325, "timeout (1 sec)"=200.0) -> ("error out"=w322:errorcluster, "watchdogID"=w323:u64)  [unwired: 1 in, 2 out]
            n130 = flat-sequence {
              tunnel: w311 -> [w388]
              tunnel: w312 -> [w389]
              tunnel: [w387] -> w339
              tunnel: [w386] -> w338
              tunnel: [w385] -> w337
              tunnel: [w384] -> w336
              tunnel: [w383] -> w335
              tunnel: [w382] -> w334
              tunnel: [w372] -> w327
              tunnel: w323 -> [w371]
              tunnel: w322 -> [w370]
              tunnel: [w371] -> w321
              tunnel: [w370] -> w320
              tunnel: [w404] -> w348
              tunnel: [w421] -> w347
              tunnel: [w420] -> w346
              tunnel: [w419] -> w345
              tunnel: [w412] -> w344
              tunnel: w339 -> [w418]
              tunnel: w338 -> [w417]
              tunnel: w337 -> [w416]
              tunnel: w336 -> [w415]
              tunnel: w335 -> [w414]
              tunnel: w334 -> [w413]
              tunnel: w327 -> [w410]
              tunnel: [w409] -> w326
              tunnel: w321 -> [w408]
              tunnel: w320 -> [w407]
              tunnel: [w405] -> w319
              tunnel: w348 -> [w584]
              tunnel: w347 -> [w581]
              tunnel: w346 -> [w580]
              tunnel: w345 -> [w597]
              tunnel: [w619] -> w331
              tunnel: w344 -> [w621]
              tunnel: [w612] -> w341
              tunnel: [w613] -> w343
              tunnel: [w614] -> w342
              tunnel: w326 -> [w593]
              tunnel: w319 -> [w585]
              tunnel: [w585] -> w317
              tunnel: [w584] -> w316
              frame #0 {
                n131 = local read "Offset_rueda WS 1"() -> (w365:fxp<+/-,24,-4>)
                n132 = local read "Offset_rueda WS 2"() -> (w366:fxp<+/-,24,-4>)
                n133 = local read "Frecuencia de muestreo (Hz)"() -> (w380:dbl)
                n134 = local read "Escaneos de la FIFO por canal"() -> (w369:u32)
                n135 = local read "Canal cero WS1?"() -> (w374:bool)
                n136 = local read "Count(mSec)"() -> (w373:u32)
                n137 = local read "Frecuencia de muestreo y módulo CRIO"() -> (w376:T3)
                n138 = local read "Canal cero WS2"() -> (w364:bool)
                n139 = local read "Digital?"() -> (w375:bool)
                n140 = Get Date/Time In Seconds() -> (seconds since 1Jan1904=→"Inicio pasada":timestamp)
                n141 = local read "Nº de acelerómetros"() -> (w362:i32)
                n142 = local read "Nº inductivos"() -> (w363:i32)
                n143 = xnode "Read/Write Control"("FPGA VI Reference In"=w389, "error in"=w388, "Data Rate"=w376, "Digital?"=w375, "Canal cero WS1?"=w374, "Count(mSec)"=w373, "Offset_WS1"=w365, "Offset_WS2"=w366, "Canal cero WS2?"=w364) -> ("FPGA VI Reference Out"=w379:refnum<k20>, "error out"=w378:errorcluster)
                n144 = local read "RFID LR6 on?"() -> (w367:bool)
                n145 = Add(x=w363, y=w362) -> (x+y=w368:i32)
                n146 = case shown="True" w367 {
                  tunnel: [errorcluster {"status"=FALSE, "code"=0, "source"=""} ("error out") w394] -> w372
                  frame False {
                  }
                  frame True {
                    n147 = local read "RFID_LR6_Error"() -> (w395:errorcluster)
                    n148 = call "LH6HD.vi"("error in (no error)"=w395, "Action"=enum16{"Init", "Start", "Read", "Stop", "Exit"}."Start") -> ("error out"=w394:errorcluster)  [unwired: 8 in, 1 out]
                  }
                }
                n149 = call "DMACalc.vi"("Number of Channels"=w368, "Number of Samples"=w369, "Rate (Hz)"=w380) -> ("Block Size"=w384:u32, "Time to Acquire Block (ms)"=w385:i32, "Host Buffer Size"=w390:u32)  [unwired: 6 in]
                n150 = call "Pathhorafech(SubVI)_varios.vi"("Folder path"=path "c:/Trenes", "Nº de acelerómetros"=w362, "Nº inductivos"=w363) -> ("Acel_Paths"=w358:path[])  [unwired: 1 in, 1 out]
                "Nombre de archivo" <- w358
                n151 = Index Array(array=w358) -> (element=w357:path)  [unwired: 1 in]
                n152 = for {
                  tunnel: w358 -> [w399] mode=indexing
                  tunnel: [w398] -> w383 mode=indexing
                  tunnel: [w397] -> w382
                  n153 = Open/Create/Replace File(file path (use dialog)=w399, operation (0:open)=T5."replace or create", access (0:read/write)=enum16{"read/write", "read-only", "write-only"}."read/write", disable buffering (F)=TRUE) -> (refnum out=w398:refnum<file>, error out=w397:errorcluster)  [unwired: 1 in, 2 out]
                }
                n154 = xnode "Invoke Method"("FPGA VI Reference In"=w379, "error in"=w378, "Requested Depth"=w390) -> ("FPGA VI Reference Out"=w392:refnum<k20>, "error out"=w391:errorcluster)  [unwired: 1 out]
                n155 = local read "Report"() -> (w361:string)
                n156 = Path To String(path=w357) -> (string=w355:string)
                n157 = Concatenate Strings("\nFile created: ", w355, "\n", w361) -> (w360:string)
                n158 = xnode "Invoke Method"("FPGA VI Reference In"=w392, "error in"=w391) -> ("FPGA VI Reference Out"=w387:refnum<k20>, "error out"=w386:errorcluster)
                n159 = local write "Report"(w360) -> ()
              }
              frame #1 {
                n160 = while "Data Acquisition" {
                  tunnel: w418 -> [w472]
                  shift-right: [w496] -> _
                  shift-left: u32 0 ("t") -> [w492]
                  tunnel: w416 -> [w497]
                  tunnel: w415 -> [w495]
                  shift-right: [w498] -> w420
                  shift-left: w417 -> [w489]
                  tunnel: [w493] -> w421
                  tunnel: w414 -> [w476]
                  tunnel: [w477] -> w419
                  shift-right: [w475] -> w412
                  shift-left: w413 -> [w485]
                  stop <- w494 stop-if-true
                  # "Detector de presencia"
                  # "Mide el tiempo de paso del tren y con ello se puede calcular\nla velocidad la unidad"
                  n161 = xnode "Invoke Method"("FPGA VI Reference In"=w472, "error in"=w489, "Number of Elements"=w492, "Timeout (ms)"=0) -> ("FPGA VI Reference Out"=w469:refnum<k20>, "error out"=w474:errorcluster, "Data"=w488:fxp<+/-,24,4>[], "Elements Remaining"=w490:u32)
                  n162 = case "Data Ready" shown="Default" w492 {
                    tunnel: w497 -> [w520 _]
                    tunnel: [w519 u32 0 ("t")] -> w496
                    tunnel: w495 -> [w521 _]
                    tunnel: w490 -> [w518 _]
                    tunnel: w488 -> [_ w543]
                    tunnel: w485 -> [w517 w542]
                    tunnel: [w517 w544] -> w475
                    tunnel: w476 -> [w516 w541]
                    tunnel: [w516 w540] -> w477
                    frame 0 {
                      # "En este caso se compara los elementos que quedan\nen la FIFO del controlador con el tamaño dell bloque\nque aparece en el panel frontal. Si el número de \nelementos en la FIFO es mayor o igual que el tamaño\n del bloque se pasa al siguiente caso y se guardan \nlos datos en un archivo. El reloj que aparece es una\nespera para no consumir recursos."
                      n163 = Greater Or Equal?(x=w518, y=w521) -> (x >= y?=w522:bool)
                      n164 = case shown="False" w522 {
                        tunnel: [u32 0 ("Block Size") w526] -> w519
                        tunnel: [w525 0 ("t")] -> w523
                        tunnel: w520 -> [w525 _]
                        tunnel: w521 -> [_ w526]
                        frame False {
                        }
                        frame True {
                        }
                      }
                      n165 = call "WaitMinTimeBetweenCall.vi"("Minimum ms between calls"=w523) -> ()  [unwired: 2 in]
                    }
                    frame Default {
                      n166 = To Single Precision Float(number=w543) -> (single precision float=w530:sgl[])
                      n167 = Decimate 1D Array(w530) -> (w536:sgl[], w539:sgl[], w538:sgl[], w537:sgl[], w535:sgl[], w534:sgl[], w533:sgl[], w532:sgl[], w531:sgl[], w528:sgl[])
                      n168 = Build Array(w536, w539, w538, w537, w535, w534, w533, w532, w531, w528) -> (w529:sgl[][])
                      n169 = for {
                        tunnel: T6."little-endian" ("byte order (0:big-endian, network order)") -> [w553]
                        shift-right: [w547] -> w544
                        shift-left: w542 -> [w548]
                        tunnel: w529 -> [w551] mode=indexing
                        tunnel: w541 -> [w550] mode=indexing
                        tunnel: [w549] -> w540 mode=indexing
                        n170 = Write to Binary File(file (use dialog)=w550, data=w551, error in=w548, 5:FALSE ("prepend array or string size? (T)"), 9:w553) -> (refnum out=w549:refnum<file>, error out=w547:errorcluster)  [unwired: 2 out]
                      }
                    }
                  }
                  n171 = xnode "Read/Write Control"("FPGA VI Reference In"=w469, "error in"=w474) -> ("FPGA VI Reference Out"=w487:refnum<k20>, "error out"=w486:errorcluster, "Parar"=w465:bool, "Nº Ruedas 1"=→"Nº Ruedas 1":i32, "NºRuedas 2"=→"NºRuedas 2":i32)
                  "Parar" <- w465
                  n172 = case shown="False" w465 {
                    tunnel: [w503 w511] -> w466
                    tunnel: [w504 0.0] -> w480
                    frame False {
                      n173 = local read "Inicio pasada"() -> (w507:timestamp)
                      n174 = Get Date/Time In Seconds() -> (seconds since 1Jan1904=w506:timestamp)
                      n175 = local read "Tiempo de adquisicion"() -> (w499:dbl)
                      n176 = To Double Precision Float(number=w506) -> (double precision float=w505:dbl)
                      n177 = To Double Precision Float(number=w507) -> (double precision float=w508:dbl)
                      n178 = Subtract(x=w505, y=w508) -> (x-y=w504:dbl)
                      "Tiempo de paso (s)" <- w504
                      n179 = local write "Tiempo"(w505) -> ()
                      n180 = local read "Boton Adquirir?"() -> (w500:bool)
                      n181 = Greater?(x=w504, y=w499) -> (0:w502:bool)
                      n182 = Select(t=w502, s=w500, f=FALSE) -> (s? t:f=w503:bool)
                    }
                    frame True {
                      n183 = local read "Tiempo"() -> (w515:dbl)
                      n184 = local read "Tiempo extra al detector de paso (s)"() -> (w510:dbl)
                      n185 = Get Date/Time In Seconds() -> (seconds since 1Jan1904=w512:timestamp)
                      n186 = To Double Precision Float(number=w512) -> (double precision float=w513:dbl)
                      n187 = Subtract(x=w513, y=w515) -> (x-y=w514:dbl)
                      n188 = Greater?(x=w514, y=w510) -> (0:w511:bool)
                    }
                  }
                  "Fin" <- w466
                  n189 = local read "Timeout ruedas"() -> (w464:dbl)
                  n190 = xnode ("CheckLate")("FPGA VI Reference In"=w487, "error in"=w486) -> ("FPGA VI Reference Out"=w471:refnum<k20>, "error out"=w482:errorcluster, "Buffer Underflow"=→"Buffer Underflow":bool, "Buffer Overflow"=w473:bool)
                  "Buffer Overflow" <- w473
                  n191 = Greater?(x=w480, y=w464) -> (0:w478:bool)
                  "Timeout ruedas" <- w478
                  n192 = call "ErrorOverFlow.vi"("Buffer Overflow"=w473) -> ("error out"=w481:errorcluster)
                  n193 = Merge Errors(w482, w481) -> (w470:errorcluster)
                  n194 = Unbundle By Name(w475) -> ("status"=w479:bool)
                  n195 = Unbundle By Name(w470) -> ("status"=w484:bool)
                  n196 = Compound Arithmetic op=OR(w484, w466, w478, w479) -> (w494:bool)
                  "result" <- w494
                  n197 = case "Flush" shown="True" w494 {
                    tunnel: [w554 w559] -> w498
                    tunnel: [w555 w558] -> w493
                    tunnel: w471 -> [w555 w557]
                    tunnel: w470 -> [w554 w556]
                    frame False {
                    }
                    frame True {
                      n198 = xnode "Invoke Method"("FPGA VI Reference In"=w557, "error in"=w556) -> ("FPGA VI Reference Out"=w558:refnum<k20>, "error out"=w559:errorcluster)
                    }
                  }
                  "Block Size" <- w495
                  "Time to Acquire Block (ms)" <- w497
                }
                n199 = call <vilib>:"Watchdog Whack.vi"("error in (no error)"=w407, "reset watchdog after expire? (F)"=TRUE, "watchdogID in"=w408) -> ("error out"=w404:errorcluster, "watchdogID out"=w405:u64)  [unwired: 2 in, 1 out]
                n200 = local read "RFID LR6 on?"() -> (w403:bool)
                n201 = case shown="True" w403 {
                  tunnel: w410 -> [w422 w428]
                  tunnel: [w422 w427] -> w409
                  frame False {
                  }
                  frame True {
                    n202 = while {
                      shift-right: [w435] -> w427
                      shift-left: w428 -> [w436]
                      shift-right: [w434] -> w425
                      shift-left: string[] [] -> [w433]
                      shift-right: [w429] -> w423
                      shift-left: i32[] [] -> [w430]
                      i -> [w431]
                      stop <- w432 stop-if-true
                      n203 = case shown="No Error" w436 {
                        selector: w436 -> [w447 _]
                        tunnel: [w446 w462] -> w435
                        tunnel: [w442 string[] []] -> w434
                        tunnel: w433 -> [w441 _]
                        tunnel: w431 -> [w440 _]
                        tunnel: w430 -> [w439 _]
                        tunnel: [w438 i32[] []] -> w429
                        frame No Error {
                          n204 = call "LH6HD.vi"("error in (no error)"=w447, "Action"=enum16{"Init", "Start", "Read", "Stop", "Exit"}."Read") -> ("error out"=w446:errorcluster, "Tag"=w443:string)  [unwired: 8 in]
                          n205 = Not Equal?(x="", y=w443) -> (x != y?=w444:bool)
                          n206 = case shown="False" w444 {
                            tunnel: w443 -> [_ w456]
                            tunnel: [w450 w455] -> w442
                            tunnel: w441 -> [w450 w454]
                            tunnel: w440 -> [_ w451]
                            tunnel: w439 -> [w449 w453]
                            tunnel: [w449 w452] -> w438
                            frame False {
                            }
                            frame True {
                              n207 = Build Array (concatenate)(w454, w456) -> (w455:string[])
                              n208 = Build Array (concatenate)(w453, w451) -> (w452:i32[])
                            }
                          }
                        }
                        frame Error {
                          n209 = local read "LR6 IP address"() -> (w459:string)
                          n210 = local read "DeviceAddress"() -> (w457:u8)
                          n211 = local read "Port LR6"() -> (w460:u16)
                          n212 = call "LH6HD.vi"("DeviceAddress"=w457, "Reader Port"=w460, "IP Address"=w459, "Action"=enum16{"Init", "Start", "Read", "Stop", "Exit"}."Init") -> ("error out"=w462:errorcluster)  [unwired: 6 in, 1 out]
                        }
                      }
                      n213 = Wait Until Next ms Multiple(millisecond multiple=u32 500) -> ()  [unwired: 1 out]
                      n214 = local read "result"() -> (w432:bool)
                      "it-LR6" <- w431
                    }
                    "TAGs LR6" <- w425
                    "it-read-LR6" <- w423
                  }
                }
              }
              frame #2 {
                # "ORGANIZAR\nTAGS AQUÍ"
                n215 = local read "RFID LR6 on?"() -> (w582:bool)
                n216 = local read "RFID NEM on?"() -> (w583:bool)
                n217 = Array Size(array=w597) -> (size(s)=w595:i32)
                n218 = local read "AURA wheel test"() -> (w563:bool)
                n219 = Decrement(x=w595) -> (x-1=w596:i32)
                n220 = case shown="True" w582 {
                  tunnel: w593 -> [w627 w633]
                  tunnel: [w627 w628] -> w592
                  frame False {
                  }
                  frame True {
                    n221 = call "LH6HD.vi"("error in (no error)"=w633, "Action"=enum16{"Init", "Start", "Read", "Stop", "Exit"}."Stop") -> ("error out"=w628:errorcluster)  [unwired: 8 in, 1 out]
                    n222 = call "Reporting_error.vi"("error out 2"=w628, "Concept"="Active RFID") -> ("Reporting"=w630:string)  [unwired: 1 in]
                    n223 = local read "Report"() -> (w631:string)
                    n224 = Concatenate Strings(w630, w631) -> (w629:string)
                    n225 = local write "Report"(w629) -> ()
                  }
                }
                n226 = case shown="True" w583 {
                  tunnel: [string[] [] ("TagArray") w640] -> w561
                  tunnel: [cluster{"TagCode":string, "FirstSeemUs":u64}[] [] ("TagData out") w639] -> w560
                  frame False {
                  }
                  frame True {
                    n227 = call "IF2_TagBuffer.vi"("Action"=enum16{"Init", "WriteTagData", "ReadTagData"}."ReadTagData") -> ("error out"=w638:errorcluster, "TagData out"=w639:cluster{"TagCode":string, "FirstSeemUs":u64}[])  [unwired: 9 in]
                    n228 = local read "connection ID"() -> (w637:refnum<k5>)
                    n229 = call "RFID_TAGS_Sort.vi"("TagData in"=w639) -> ("TagString"=w641:string, "TagArray"=w640:string[])  [unwired: 9 in]
                    n230 = call "IF2_Clear_buffer.vi"("error in (no error)"=w638, "TCP Network Connection in"=w637) -> ()  [unwired: 8 in, 2 out]
                    n231 = call "Reporting_error.vi"("error out 2"=w638, "Concept explanation"=w641, "Concept"="Passive RFID") -> ("Reporting"=w644:string)
                    n232 = local read "Report"() -> (w645:string)
                    n233 = Concatenate Strings(w644, w645) -> (w643:string)
                    n234 = local write "Report"(w643) -> ()
                  }
                }
                "TAGs HEX" <- w561
                n235 = Index Array(array=w597, index=w596) -> (element=w605:refnum<file>)
                n236 = local write "result"(FALSE ("result")) -> ()
                n237 = xnode "Read/Write Control"("FPGA VI Reference In"=w581, "error in"=w580) -> ("FPGA VI Reference Out"=w618:refnum<k20>, "error out"=w578:errorcluster, "Chassis Temperature"=w626:i16)
                n238 = local read "TAGs LR6"() -> (w565:string[])
                n239 = Select(t=string[] ["A0000000000000000TESTNEM7", "A0000000000000000TESTNEM8"], s=w563, f=w565) -> (s? t:f=w562:string[])
                n240 = Divide(x=w626, y=4.0) -> (x/y=w574:dbl)
                "Temperatura (ºC)" <- w574
                n241 = local read "Tiempo de paso (s)"() -> (w616:dbl)
                n242 = for {
                  tunnel: w562 -> [w649] mode=indexing
                  tunnel: [w647] -> w586 mode=indexing
                  n243 = Search and Replace String(input string=w649, search string="00") -> (result string=w647:string)  [unwired: 6 in, 3 out]
                }
                n244 = local write "RFID_LR6_Error"(w592) -> ()
                n245 = Index Array(array=w561) -> (element=w591:string)  [unwired: 1 in]
                n246 = local read "Nº Ruedas 1"() -> (w572:i32)
                n247 = local read "NºRuedas 2"() -> (w576:i32)
                n248 = Not Equal?(x=w591, y="" ("delimiter (\\t)")) -> (x != y?=w589:bool)
                "Plataformas?" <- w589
                n249 = Multiply(x=w616, y=1000.0) -> (x*y=w573:dbl)
                n250 = case shown="True" w589 {
                  tunnel: w586 -> [w650 w657]
                  tunnel: [w650 w656] -> w575
                  tunnel: w561 -> [_ _]
                  tunnel: w560 -> [_ w652]
                  frame False {
                  }
                  frame True {
                    n251 = local read "Tiempo de paso (s)"() -> (w655:dbl)
                    n252 = local read "Tabla_flota"() -> (w653:string[][])
                    n253 = local read "Inicio pasada"() -> (w654:timestamp)
                    n254 = local read "RFID_status"() -> (w651:path)
                    n255 = call "Union_TAGs_RFIDs.vi"("TAGs LR6"=w657) -> ()  [unwired: 1 in, 1 out]
                    n256 = call "write_tag_status.vi"("Inicio pasada"=w654, "Tabla_flota"=w653, "TagData in"=w652, "file path (use dialog)"=w651) -> ()  [unwired: 7 in]
                    n257 = call "TagNormalizaction.vi"("Inicio pasada"=w654, "Tiempo de paso (s)"=w655, "TagData in"=w652, "Tabla_flota"=w653) -> ("Normalized Tags"=w656:string[])  [unwired: 7 in]
                  }
                }
                "TAGs" <- w575
                n258 = Build Array(w574, w573, w572, w576) -> (w577:dbl[])
                n259 = Build Array(w574, w573, w572) -> (w571:dbl[])
                n260 = local read "Direccion 0?"() -> (w570:bool)
                n261 = local read "Nombre de archivo"() -> (w604:path[])
                n262 = Bundle("error out"=w578, w577, "Normalized Tags"=w575, "Direccion 0?"=w570) -> (w569:T11)  [unwired: 1 in]
                n263 = for {
                  shift-right: [w663] -> w610
                  shift-left: string[] [] -> [w662]
                  tunnel: w575 -> [w661] mode=indexing
                  n264 = Insert Into Array(array=w662, new element=w661) -> (w663:string[])  [unwired: 1 in]
                }
                n265 = xnode "Read/Write Control"("FPGA VI Reference In"=w618, "error in"=w578, "Stop"=TRUE ("stop")) -> ("FPGA VI Reference Out"=w607:refnum<k20>, "error out"=w606:errorcluster)
                n266 = call "Reporting_acqu.vi"("output cluster"=w569, "address repoting"=path "C:/Reporting/Reporting_adqu.txt" ("file (use dialog)")) -> ("Reporting"=w566:string)  [unwired: 1 in]
                n267 = Delete From Array(array=w604) -> (deleted portion=w603:path)  [unwired: 2 in, 1 out]
                n268 = local read "Report"() -> (w567:string)
                n269 = To Single Precision Float(number=w571) -> (single precision float=w624:sgl[])
                n270 = Path To String(path=w603) -> (string=w609:string)
                n271 = Concatenate Strings(w566, w567) -> (w568:string)
                n272 = Write to Binary File(file (use dialog)=w605, data=w624, error in=w621, 5:FALSE ("prepend array or string size? (T)"), 9:T6."little-endian" ("byte order (0:big-endian, network order)")) -> (error out=w602:errorcluster)  [unwired: 3 out]
                n273 = xnode "Invoke Method"("FPGA VI Reference In"=w607, "error in"=w606) -> ("FPGA VI Reference Out"=w614:refnum<k20>, "error out"=w613:errorcluster)
                n274 = local read "Timeout ruedas"() -> (w617:bool)
                n275 = local write "Report"(w568) -> ()
                n276 = Build Array (concatenate)(w609, w610) -> (w587:string[])
                n277 = local read "TAGS leidos"() -> (w598:path)
                n278 = for {
                  shift-right: [w660] -> w612
                  shift-left: w602 -> [w659]
                  tunnel: w597 -> [w658] mode=indexing
                  n279 = Close File(refnum=w658, error in=w659) -> (error out=w660:errorcluster)  [unwired: 1 out]
                }
                n280 = call-poly <vilib>:"Write Delimited Spreadsheet.vi"("file path (dialog if empty)"=w598, "1D data"=w587, "append to file? (F)"=TRUE ("transpose? (no:F)"), "transpose? (F)"=TRUE ("append to file? (new file:F)"), "delimiter (\\t)"=";" ("delimiter (\\t)")) -> ()  [unwired: 9 in, 2 out]
                n281 = Select(t="TEST", s=w617, f="Procesado") -> (s? t:f=w619:string)
              }
            }
            n282 = call <vilib>:"Watchdog Clear.vi"("error in (no error)"=w316, "watchdogID in"=w317) -> ("error out"=w318:errorcluster)  [unwired: 5 in]
            n283 = Unbundle By Name(w343) -> ("status"=w332:bool)
            n284 = Unbundle By Name(w341) -> ("status"=w333:bool)
            n285 = Merge Errors(w341, w318) -> (w340:errorcluster)
            n286 = Compound Arithmetic op=OR(w332, w333) -> (w330:bool)
            n287 = Select(t="TEST", s=w330, f=w331) -> (s? t:f=w328:string)
          }
          frame "Procesado" {
            n288 = local read "Watchdog config"() -> (w675:T2)
            n289 = flat-sequence {
              tunnel: w669 -> [w688]
              tunnel: [w688] -> w668
              tunnel: w667 -> [w684]
              tunnel: [w684] -> w666
              frame #0 {
                n290 = local read "Report"() -> (w685:string)
                n291 = call "Reporting_datetime.vi"() -> ("String"=w683:string)  [unwired: 11 in]
                n292 = Concatenate Strings(w683, "\nSTATUS: PROCESSING\nProcessing the measurement\n\n", w685) -> (w687:string)
                n293 = local write "Report"(w687) -> ()
              }
            }
            n294 = call <vilib>:"Watchdog Configure.vi"("error in (no error)"=w678, "expiration actions"=w675, "timeout (1 sec)"=300.0) -> ("error out"=w677:errorcluster, "watchdogID"=w674:u64)  [unwired: 1 in, 2 out]
            n295 = flat-sequence {
              tunnel: w677 -> [w695]
              tunnel: w674 -> [w691]
              tunnel: [w690] -> w673
              tunnel: [w689] -> w672
              tunnel: [w906] -> w671
              tunnel: w673 -> [w906]
              tunnel: [w905] -> w670
              tunnel: w672 -> [w905]
              frame #0 {
                n296 = flat-sequence {
                  tunnel: [w767] -> w697
                  tunnel: [w753] -> w696
                  tunnel: w695 -> [w734]
                  tunnel: [w716] -> w692
                  tunnel: [w755] -> w694
                  tunnel: [w707] -> w693
                  tunnel: w691 -> [w735]
                  tunnel: [w732] -> w690
                  tunnel: [w731] -> w689
                  frame #0 {
                    n297 = local read "AURA wheel test"() -> (w705:bool)
                    n298 = case shown="False" w705 {
                      tunnel: [w770 w771] -> w704
                      tunnel: [w769 path[] [path "c:/Trenes_prueba/A_0_TEST.bin", path "c:/Trenes_prueba/A_1_TEST.bin", path "c:/Trenes_prueba/A_2_TEST.bin", path "c:/Trenes_prueba/A_3_TEST.bin", path "c:/Trenes_prueba/A_4_TEST.bin", path "c:/Trenes_prueba/A_5_TEST.bin", path "c:/Trenes_prueba/A_6_TEST.bin", path "c:/Trenes_prueba/A_7_TEST.bin", path "c:/Trenes_prueba/I_0_TEST.bin", path "c:/Trenes_prueba/I_1_TEST.bin"]] -> w703
                      frame False {
                        n299 = local read "Nombre de archivo"() -> (w769:path[])
                        n300 = local read "TAGs"() -> (w770:string[])
                      }
                      frame True {
                        w771 = string[] ["A0000000000000000TESTNEM7", "A0000000000000000TESTNEM8"]
                        n301 = local write "TAGs LR6"(w771) -> ()
                      }
                    }
                    n302 = local read "Tabla_flota"() -> (w752:string[][])
                    n303 = call <vilib>:"Watchdog Whack.vi"("error in (no error)"=w734, "reset watchdog after expire? (F)"=TRUE, "watchdogID in"=w735) -> ("error out"=w731:errorcluster, "watchdogID out"=w732:u64)  [unwired: 2 in, 1 out]
                    n304 = local read "Puntos medios de las ventanas"() -> (w754:dbl[][])
                    n305 = call "Series_ejes_flota.vi"("Tabla_flota"=w752, "Tags"=w704) -> ("Nº Ejes"=w729:i32[], "Series del convoy"=w746:string[])  [unwired: 2 in, 1 out]
                    "Nº Ejes" <- w729
                    n306 = Array Size(array=w703) -> (size(s)=w761:i32)
                    n307 = Add Array Elements(numeric array=w729) -> (sum=w715:i32)
                    "Ejes_convoy" <- w715
                    n308 = Subtract(x=w761, y=2 ("length")) -> (x-y=w763:i32)
                    n309 = Array Size(array=w746) -> (size(s)=→"Nº UTs":i32)
                    n310 = local read "Series_flota"() -> (w751:string[])
                    n311 = Delete From Array(array=w703, length=2, index=w763) -> (deleted portion=w736:path[], array with subset deleted=w755:path[])
                    n312 = Index Array(array=w736) -> (element #2=w730:path)  [unwired: 2 in, 1 out]
                    n313 = call "Distancias_ejes_convoy.vi"("Series_flota1"=w746, "Ejes_UT"=w729, "Puntos medios de las ventanas"=w754, "Series_flota"=w751) -> ("Distancias_entre_ejes_convoy"=w753:dbl[])  [unwired: 1 in]
                    n314 = Read from Binary File(5:sgl 0.0, 9:T6."little-endian" ("byte order (0:big-endian, network order)"), 10:-1 ("count (1)"), 11:w730) -> (0:w759:errorcluster, 2:w738:sgl[], 3:w760:refnum<file>)  [unwired: 1 in, 2 out]
                    n315 = local read "Frecuencia de muestreo (Hz)"() -> (w720:dbl)
                    n316 = local read "Offset_rueda WS 2"() -> (w721:fxp<+/-,24,-4>)
                    n317 = local read "it-LR6"() -> (w741:i32)
                    n318 = local read "it-read-LR6"() -> (w742:i32[])
                    n319 = local read "Plataformas?"() -> (w740:bool)
                    n320 = local read "TAGs"() -> (w744:string[])
                    n321 = local read "TAGs LR6"() -> (w743:string[])
                    n322 = Close File(refnum=w760, error in=w759) -> (error out=w699:errorcluster)  [unwired: 1 out]
                    n323 = Array Size(array=w738) -> (size(s)=w750:i32)
                    n324 = Subtract(x=w750, y=3 ("length")) -> (x-y=w748:i32)
                    n325 = Delete From Array(array=w738, length=3, index=w748) -> (array with subset deleted=w727:sgl[])  [unwired: 1 out]
                    n326 = call "TAGs_AURAwheel_TAGM_NEM.vi"("Nº Ejes"=w729, "TAGs"=w744, "Ejes_convoy"=w715, "it-LR6"=w741, "TAGs LR6"=w743, "it-read-LR6"=w742, "Plataformas?"=w740) -> ("TAGS_AURA"=→"TAGs_AURAwheel":string[][])  [unwired: 1 in]
                    n327 = call "Analogico_digital.vi"("Array"=w727, "Offset WS"=w721, "Frecuencia muestreo"=w720) -> ("array w/ subset deleted"=w722:sgl[], "Tiempo\npaso"=w719:dbl)  [unwired: 6 in]
                    n328 = call "Puntos medio de pulso.vi"("DI Inductivo"=w722) -> ("Puntos"=w767:sgl[], "Número de ejes"=w709:i32)  [unwired: 1 in]
                    "Número de ejes detectados" <- w709
                    n329 = disable-structure shown="Enabled" {
                      disable-tunnel: w727 -> [w779 w782]
                      disable-tunnel: [FALSE ("element") TRUE ("element")] -> w724
                      disable-tunnel: [w773 w781] -> w723
                      frame Disabled {
                        n330 = Equal?(x=w779, y=0.0) -> (x = y?=w776:bool[])
                        n331 = Equal?(x=w779, y=1.0) -> (x = y?=w777:bool[])
                        n332 = Or(x=w776, y=w777) -> (x .or. y?=w773:bool[])
                      }
                      frame Enabled {
                        n333 = Greater?(x=w782, y=0.1) -> (0:w781:bool[])
                      }
                    }
                    n334 = Decrement(x=w709) -> (x-1=w766:i32)
                    n335 = call "Reporting_error.vi"("error out 2"=w699, "Concept"="Measurement reading") -> ("Reporting"=w701:string)  [unwired: 1 in]
                    n336 = Get Volume Info(11:path "c:/" ("path")) -> (1:w710:i64)  [unwired: 1 in, 5 out]
                    "Disco Duro Disponible (bytes)" <- w710
                    n337 = local read "Report"() -> (w702:string)
                    n338 = call "Calculo_Velocidad.vi"("Tiempo de paso (s)"=w719, "Ejes"=w766, "Puntos iniciales de las ventanas"=w753) -> ("V (m/s)"=→"V (m/s)":dbl, "Longitud de la unidad"=→"Longitud de la unidad":dbl)
                    n339 = Concatenate Strings(w701, w702) -> (w700:string)
                    n340 = Equal?(x=w715, y=w709) -> (x = y?=w707:bool)
                    n341 = Not Equal?(x=w709, y=0) -> (x != y?=w706:bool)
                    n342 = Search 1D Array(1D array=w723, element=w724) -> (index of element=w725:i32)  [unwired: 1 in]
                    n343 = local write "Report"(w700) -> ()
                    n344 = Build Array(w715, w709, w710) -> (w714:i64[])
                    n345 = Equal?(x=w725, y=-1) -> (x = y?=w728:bool)
                    n346 = Compound Arithmetic op=AND(w707, w706, w728) -> (w716:bool)
                    "Archivo\nvalido?" <- w716
                    n347 = Bundle(w714, w716) -> (w712:cluster{i64[], bool})  [unwired: 1 in]
                    n348 = call "Reporting_proc.vi"("output cluster 2"=w712, "address repoting"=path "C:/Reporting/Reporting_proc.txt" ("file (use dialog)")) -> ("Reporting"=w711:string)  [unwired: 1 in]
                    n349 = local read "Report"() -> (w717:string)
                    n350 = Concatenate Strings(w711, w717) -> (w718:string)
                    n351 = local write "Report"(w718) -> ()
                  }
                }
                n352 = case shown="True" w692 {
                  tunnel: w697 -> [_ w817]
                  tunnel: w696 -> [_ w815]
                  tunnel: w694 -> [_ w816]
                  tunnel: w693 -> [w784 _]
                  frame False {
                    n353 = local read "Nombre de archivo"() -> (w785:path[])
                    n354 = for {
                      tunnel: w785 -> [w787] mode=indexing
                      tunnel: w784 -> [w786]
                      n355 = flat-sequence {
                        tunnel: w787 -> [w797]
                        tunnel: [w797] -> w790
                        tunnel: [w796] -> w789
                        tunnel: w786 -> [w795]
                        tunnel: w790 -> [w804]
                        tunnel: [w803] -> w788
                        tunnel: w789 -> [w803]
                        tunnel: w788 -> [w806]
                        frame #0 {
                          w796 = path "c:/Est_Adq.csv" ("file path (use dialog)")
                          n356 = Path To String(path=w797) -> (string=w798:string)
                          n357 = Select(t="Nº Ejes detectados WS diferente a Nº Ejes TAGs" ("delimiter (\\t)"), s=w795, f="La señal del inductivo no es digital" ("delimiter (\\t)")) -> (s? t:f=w792:string)
                          n358 = Build Array(w798, w792) -> (w791:string[])
                          n359 = call-poly <vilib>:"Write Delimited Spreadsheet.vi"("file path (dialog if empty)"=w796, "1D data"=w791, "append to file? (F)"=FALSE ("transpose? (no:F)"), "transpose? (F)"=TRUE ("append to file? (new file:F)"), "delimiter (\\t)"=";" ("delimiter (\\t)")) -> ()  [unwired: 9 in, 2 out]
                        }
                        frame #1 {
                          n360 = local read "Borrar archivos\nadquisicion con error"() -> (w802:bool)
                          n361 = case shown="True" w802 {
                            tunnel: w804 -> [_ w805]
                            frame False {
                            }
                            frame True {
                              n362 = Delete(path (use dialog)=w805) -> ()  [unwired: 1 in, 6 out]
                            }
                          }
                        }
                        frame #2 {
                          n363 = File/Directory Info(path=w806) -> (size=w809:i64)  [unwired: 1 in, 6 out]
                          n364 = Greater?(x=w809, y=i64 1000000) -> (0:w807:bool)
                          n365 = case shown="True" w807 {
                            tunnel: w806 -> [_ w810]
                            frame False {
                            }
                            frame True {
                              n366 = Delete(path (use dialog)=w810) -> ()  [unwired: 4 in, 3 out]
                            }
                          }
                        }
                      }
                    }
                  }
                  frame True {
                    n367 = flat-sequence {
                      tunnel: w817 -> [w894]
                      tunnel: w816 -> [w891]
                      tunnel: w815 -> [w895]
                      tunnel: [w878] -> w814
                      frame #0 {
                        # "SALIDA \n\nMáximos por rueda inductivo"
                        # "8 acelerómetros"
                        # "Velocidad"
                        n368 = local read "Frecuencia de muestreo (Hz)"() -> (w893:dbl)
                        n369 = local read "Distancia de acelerómetros"() -> (w883:dbl[])
                        n370 = local read "Parámetros acelerómetros"() -> (w890:dbl[])
                        n371 = local read "Número de ejes detectados"() -> (w889:i32)
                        n372 = local read "Distancias generales"() -> (w888:dbl[])
                        n373 = local read "dt RMS"() -> (w892:dbl)
                        n374 = local read "Direccion 0?"() -> (w880:bool)
                        n375 = Index Array(array=w888, index=1) -> (element=w886:dbl)
                        n376 = Select(t=0.0, s=w880, f=w886) -> (s? t:f=w884:dbl)
                        n377 = Subtract(x=w884, y=w883) -> (x-y=w882:dbl[])
                        n378 = Absolute Value(x=w882) -> (abs(x)=w881:dbl[])
                        n379 = call "Procesado_aRMS_BIdirecc.vi"("Paths_canales_aRMS"=w891, "Ejes Procesados"=w889, "Distancias\nacelerometros"=w881, "Distancias generales (m)"=w888, "Distancias centrales de las ruedas\n               configuración (m)"=w895, "Frecuencia de muestreo"=w893, "Parámetros acelerómetros"=w890, "dt RMS 2"=w892, "Puntos"=w894) -> ("Max RMS Ruedas"=w879:dbl[][])  [unwired: 2 in]
                        n380 = Transpose 2D Array(2D array=w879) -> (transposed array=w878:dbl[][])
                        "Max RMS Ruedas" <- w878
                        n381 = call "Reporting_proc_RMS.vi"("Max RMS Ruedas"=w878) -> ("String"=w876:string)
                        n382 = local read "Report"() -> (w877:string)
                        n383 = Concatenate Strings(w876, w877) -> (w875:string)
                        n384 = local write "Report"(w875) -> ()
                      }
                    }
                    n385 = local read "Use Aura?"() -> (w813:bool)
                    n386 = local read "TAGs_AURAwheel"() -> (w812:string[][])
                    n387 = local read "Nº Ejes"() -> (w811:i32[])
                    n388 = for {
                      tunnel: w813 -> [w821]
                      tunnel: w812 -> [w820] mode=indexing
                      shift-right: [w819] -> _
                      shift-left: w814 -> [w822]
                      tunnel: w811 -> [w818] mode=indexing
                      # "dev.api.aurawheel.com"
                      n389 = case shown="True" w821 {
                        tunnel: w822 -> [w823 w842]
                        tunnel: w820 -> [_ w843]
                        tunnel: [w823 w841] -> w819
                        tunnel: w818 -> [_ w839]
                        frame False {
                        }
                        frame True {
                          w827 = "\n"
                          w850 = cluster{"status":string} {"status"=""}
                          n390 = local read "Parametros AuraWheel"() -> (w874:string[])
                          n391 = Delete From Array(array=w842, length=w839, index (row)=0) -> (deleted portion=w838:dbl[][], array with subset deleted=w841:dbl[][])  [unwired: 1 in]
                          n392 = Get Date/Time In Seconds() -> (seconds since 1Jan1904=w871:timestamp)
                          n393 = Format Date/Time String(time format string (%c)="%H:%M:%S%3u", seconds (now)=w871) -> (date/time string=w869:string)  [unwired: 1 in]
                          n394 = Get Date/Time In Seconds() -> (seconds since 1Jan1904=w846:timestamp)
                          n395 = Scan From String(format string="%d:%d:%f", input string=w869) -> (output 1=w866:i32, output 2=w865:i32, output 3=w863:dbl)  [unwired: 5 in, 3 out]
                          n396 = local read "V (m/s)"() -> (w834:dbl)
                          n397 = local read "Temperatura (ºC)"() -> (w844:dbl)
                          n398 = Multiply(x=w834, y=3.6) -> (x*y=w832:dbl)
                          n399 = Multiply(x=w863, y=1000.0) -> (x*y=w859:dbl)
                          n400 = call "Time_to_ms.vi"("seconds since 1Jan1904"=w846) -> ("Numeric"=w845:dbl)  [unwired: 1 in]
                          n401 = Multiply(x=w865, y=60000) -> (x*y=w860:i32)
                          n402 = Multiply(x=3600000, y=w866) -> (x*y=w861:i32)
                          n403 = Index Array(array=w874) -> (element #1=w837:string, element #2=w836:string, element #3=w835:string)  [unwired: 3 in]
                          n404 = call "aw_WRDCluster_8acel.vi"("Array TAGs"=w843, "Max RMS Ruedas"=w838, "TimeStamp"=w845, "p_sp"=w832, "p_tp"=w844) -> ("JSON cluster"=w872:T12)  [unwired: 1 in]
                          n405 = Compound Arithmetic op=ADD(w861, w860, w859) -> (w858:dbl)
                          n406 = To Variant(anything=w872) -> (Variant=w855:variant)
                          n407 = To Unsigned Long Integer(number=w858) -> (unsigned 32bit integer=w857:u32)
                          n408 = call "gjson_Create.vi"("JSON Object in"=w855) -> ("error out"=w853:errorcluster, "JSON String Out"=w854:string)  [unwired: 9 in]
                          n409 = Number To Decimal String(number=w857) -> (decimal integer string=w856:string)  [unwired: 1 in]
                          n410 = To Variant(anything=w850) -> (Variant=w849:variant)
                          n411 = call "aw_SendData.vi"("pwd"=w837, "x-nem-datetime"=w856, "User"=w836, "error in"=w853, "JSON Object"=w854, "URL"=w835) -> ("error out"=w851:errorcluster, "Response JSON"=w852:string, "Response headers"=w828:string)  [unwired: 3 in]
                          "Response headers" <- w828
                          n412 = call "gjson_Parse.vi"("error in"=w851, "JSON String In"=w852, "JSON Cluster"=w849) -> ("error out"=w847:errorcluster, "JSON Cluster Out"=w848:variant)  [unwired: 7 in]
                          n413 = Variant To Data(error in=w847, type=w850, Variant=w848) -> (data=→"data":cluster{"status":string}, error out=w829:errorcluster)
                          "error AURA" <- w829
                          n414 = local read "Report"() -> (w825:string)
                          n415 = call "Reporting_error.vi"("error out 2"=w829, "Concept"="A.U.R.A. Wheel Connection") -> ("Reporting"=w830:string)  [unwired: 1 in]
                          n416 = Concatenate Strings(w830, w827, w827, w828, w827) -> (w826:string)
                          "Report_AURA" <- w826
                          n417 = Concatenate Strings(w826, w825) -> (w824:string)
                          n418 = local write "Report"(w824) -> ()
                        }
                      }
                    }
                  }
                }
              }
              frame #1 {
                n419 = local read "Archivo\nvalido?"() -> (w902:bool)
                n420 = local read "Bytes libre despues de borrar"() -> (w903:u32)
                n421 = local read "Report_AURA"() -> (w899:string)
                n422 = local read "Max archivos"() -> (w900:u32)
                n423 = local read "Path LOG"() -> (w901:path)
                n424 = local read "LOG.txt"() -> (w896:path)
                n425 = local read "Report"() -> (w898:string)
                n426 = local read "Bytes min libre"() -> (w904:u32)
                n427 = local read "TAGS leidos"() -> (w907:path)
                n428 = File/Directory Info(path=w907) -> (size=w910:i64)  [unwired: 1 in, 6 out]
                n429 = case shown="True" w902 {
                  frame False {
                  }
                  frame True {
                    n430 = local read "Nombre de archivo"() -> (w912:path[])
                    n431 = call "Comprimir_a_1_archivo.vi"("Acel_paths"=w912) -> ("path_Pasada"=→"created path":path)
                  }
                }
                n432 = Greater?(x=w910, y=i64 1000000) -> (0:w908:bool)
                n433 = case shown="True" w908 {
                  tunnel: w907 -> [_ w913]
                  frame False {
                  }
                  frame True {
                    n434 = Delete(path (use dialog)=w913) -> ()  [unwired: 4 in, 3 out]
                  }
                }
                n435 = call "BORRADO_MEJORADO_Gonzalo.vi"("Bytes LIBRE OK"=w903, "Bytes Minimo de Memoria libre"=w904) -> ()  [unwired: 10 in]
                n436 = call "Saving_LOG.vi"("Path"=w896, "Report"=w898, "Report AURA"=w899, "Path Carpeta"=w901, "Nº Archivos Max"=w900) -> ("Report"=w897:string)  [unwired: 9 in, 1 out]
                n437 = local write "Report"(w897) -> ()
              }
            }
            n438 = call <vilib>:"Watchdog Clear.vi"("error in (no error)"=w670, "watchdogID in"=w671) -> ("error out"=w664:errorcluster)  [unwired: 5 in]
            n439 = Merge Errors(w666, w664) -> (w682:errorcluster)
            n440 = Unbundle By Name(w682) -> ("status"=w680:bool)
            n441 = Select(t="TEST", s=w680, f="Espera") -> (s? t:f=w679:string)
          }
          frame "TEST" {
            n442 = flat-sequence {
              tunnel: [w929] -> w916
              tunnel: w918 -> [w929]
              frame #0 {
                n443 = local read "Report"() -> (w930:string)
                n444 = call "Reporting_datetime.vi"() -> ("String"=w928:string)  [unwired: 11 in]
                n445 = Concatenate Strings(w928, "\nSTATUS: ERROR TEST\n\n", w930) -> (w932:string)
                n446 = local write "Report"(w932) -> ()
              }
            }
            n447 = local read "Watchdog config"() -> (w923:T2)
            n448 = Merge Errors(w916, w914) -> (w915:errorcluster)
            n449 = call <vilib>:"Watchdog Configure.vi"("error in (no error)"=w914, "expiration actions"=w923, "timeout (1 sec)"=200.0) -> ("error out"=w924:errorcluster, "watchdogID"=w921:u64)  [unwired: 1 in, 2 out]
            n450 = flat-sequence {
              tunnel: [w942] -> w927
              tunnel: w924 -> [w937]
              tunnel: w915 -> [w955]
              tunnel: [w938] -> w925
              tunnel: w921 -> [w936]
              tunnel: [w935] -> w920
              tunnel: [w934] -> w919
              frame #0 {
                n451 = Get Date/Time In Seconds() -> (seconds since 1Jan1904=w949:timestamp)
                n452 = local read "Ultimo TEST"() -> (w950:timestamp)
                n453 = To Double Precision Float(number=w949) -> (double precision float=w951:dbl)
                n454 = Subtract(x=w951, y=3600.0) -> (x-y=w953:dbl)
                n455 = To Time Stamp(1:w953) -> (0:w954:timestamp)
                n456 = call <vilib>:"Watchdog Whack.vi"("error in (no error)"=w937, "reset watchdog after expire? (F)"=TRUE, "watchdogID in"=w936) -> ("error out"=w934:errorcluster, "watchdogID out"=w935:u64)  [unwired: 2 in, 1 out]
                n457 = In Range and Coerce(upper limit=w949, x=w950, lower limit=w954) -> (In Range?=w948:bool)  [unwired: 1 out]
                n458 = case shown="False" w948 {
                  tunnel: w955 -> [w965 w989]
                  tunnel: [w965 w989] -> w938
                  frame False {
                    n459 = local read "Timeout ruedas"() -> (w966:bool)
                    n460 = local read "Aviso no detección"() -> (w969:string)
                    n461 = local read "Aviso temperatura"() -> (w968:string)
                    n462 = case shown="True" w966 {
                      selector: w966 -> [_ w986]
                      tunnel: ["\r" w987] -> w964
                      frame False {
                      }
                      frame True {
                        w976 = "\n"
                        n463 = local read "Nº Ruedas 1"() -> (w983:i32)
                        n464 = local read "NºRuedas 2"() -> (w978:i32)
                        n465 = call "ErrorRuedas.vi"("Buffer Overflow"=w986) -> ("error out"=w988:errorcluster)
                        n466 = Number To Decimal String(number=w983) -> (decimal integer string=w981:string)  [unwired: 1 in]
                        n467 = Number To Decimal String(number=w978) -> (decimal integer string=w977:string)  [unwired: 1 in]
                        n468 = Concatenate Strings("Error Wheel sensors", "\n", "WS1 (wheels):", w981, w976, "WS2 (wheels):", w977, w976) -> (w979:string)
                        n469 = call "Error.vi"("Error con..."=w979, "error comunicacion 2"=w988) -> ("String"=w987:string)
                      }
                    }
                    n470 = local read "DC OK"() -> (w967:string)
                    n471 = call "Cabecera.vi"() -> ("String"=w974:string)
                    n472 = call "Adquisicion.vi"("Aviso no detección"=w969) -> ("String"=w973:string)
                    n473 = call "Temperatura.vi"("Aviso temperatura"=w968) -> ("String"=w972:string)
                    n474 = call "Fuente.vi"("DC OK"=w967) -> ("String"=w971:string)
                    n475 = call "FPGA.vi"("error out"=w965) -> ("String"=w970:string)
                    n476 = Get Date/Time In Seconds() -> (seconds since 1Jan1904=→"Ultimo TEST":timestamp)
                    n477 = Concatenate Strings(w974, w973, w972, w971, w970, w964) -> (w958:string)
                    n478 = local read "Report"() -> (w957:string)
                    n479 = Concatenate Strings(w958, w957) -> (w959:string)
                    n480 = local read "Max archivos"() -> (w960:u32)
                    n481 = local read "Path LOG"() -> (w963:path)
                    n482 = local read "LOG.txt"() -> (w961:path)
                    n483 = call "Saving_LOG.vi"("Path"=w961, "Report"=w959, "Report AURA"=w958, "Path Carpeta"=w963, "Nº Archivos Max"=w960) -> ("Report"=w962:string)  [unwired: 9 in, 1 out]
                    n484 = local write "Report"(w962) -> ()
                  }
                  frame True {
                  }
                }
                n485 = local read "Fallo fotocelula"() -> (w941:bool)
                n486 = local read "T fuera rango"() -> (w947:bool)
                n487 = Unbundle By Name(w938) -> ("status"=w939:bool)
                n488 = Compound Arithmetic op=OR(w939, w941) -> (w940:bool)
                n489 = local write "Reset del controlador"(w940) -> ()
                n490 = Select(t="UPS", s=w947, f="Espera") -> (s? t:f=w944:string)
                n491 = Select(t="Configuracion", s=w940, f=w944) -> (s? t:f=w942:string)
              }
            }
            n492 = call <vilib>:"Watchdog Clear.vi"("error in (no error)"=w919, "watchdogID in"=w920) -> ("error out"=w917:errorcluster)  [unwired: 5 in]
          }
          frame "Calibracion" {
            n493 = flat-sequence {
              tunnel: w1005 -> [w1790]
              tunnel: w1004 -> [w1789]
              tunnel: [w1790] -> w1003
              tunnel: [w1789] -> w1002
              frame #0 {
                n494 = local read "Report"() -> (w1786:string)
                n495 = call "Reporting_datetime.vi"() -> ("String"=w1785:string)  [unwired: 11 in]
                n496 = Concatenate Strings(w1785, "\nSTATUS: CALIBRATION\n\n\n", w1786) -> (w1788:string)
                n497 = local write "Report"(w1788) -> ()
              }
            }
            n498 = for {
              N: 5 -> [_]
              shift-right: [w1044] -> w996
              shift-left: w1003 -> [w1046]
              shift-right: [w1043] -> w992
              shift-left: w1002 -> [w1045]
              shift-right: [w1041] -> _
              shift-left: "Adquisicion" ("element") -> [w1042]
              shift-right: [w1040] -> _
              shift-left: _ -> [w1038]
              shift-right: [w1036] -> w991
              shift-left: "" -> [w1035]
              i -> [w1034]
              stop <- w1039 stop-if-true
              n499 = case shown="\"Adquisicion\", Default" w1042 {
                tunnel: w1046 -> [w1054 w1284 w1489 w1651 w1736]
                tunnel: w1045 -> [w1053 w1283 w1488 w1650 w1735]
                tunnel: [w1052 w1284 w1489 w1651 w1736] -> w1044
                tunnel: [w1051 w1283 w1488 w1650 w1735] -> w1043
                tunnel: ["Acel_calib" ("Concept") "Acel_frequency" ("Concept") "Acel_noise" ("Concept") "Acel_result" ("Concept") "Adquisicion" ("Concept")] -> w1041
                tunnel: [sgl[][] [] w1280 w1487 w1649 sgl[][] []] -> w1040
                tunnel: [TRUE w1279 w1486 w1646 FALSE] -> w1033
                tunnel: w1038 -> [_ _ w1477 w1652 w1746]
                tunnel: ["\n" w1277 w1484 w1642 w1734] -> w1037
                frame "Adquisicion", Default {
                  n500 = flat-sequence {
                    tunnel: w1053 -> [w1076]
                    tunnel: w1054 -> [w1077]
                    tunnel: [w1077] -> w1057
                    tunnel: [w1076] -> w1056
                    tunnel: [w1060] -> w1055
                    tunnel: w1057 -> [w1089]
                    tunnel: w1056 -> [w1088]
                    tunnel: w1055 -> [w1085]
                    tunnel: [w1087] -> w1052
                    tunnel: [w1086] -> w1051
                    frame #0 {
                      w1072 = "Calibration" ("element")
                      w1071 = "c"
                      n501 = Format Date/Time String(time format string (%c)="%Y-%m-%d-%H-%M-%S") -> (date/time string=w1063:string)  [unwired: 2 in]
                      n502 = for {
                        N: 1 -> [_]
                        shift-right: [w1078] -> w1058
                        shift-left: _ -> [w1079]
                        n503 = Add(x=w1079, y=0.001) -> (x+y=w1078:dbl)
                      }
                      n504 = Number To Fractional String(number=w1058) -> (F-format string=w1067:string)  [unwired: 3 out]
                      n505 = Search and Replace String(input string=w1067, search string="." ("replace string (\"\")")) -> (result string=w1065:string)  [unwired: 1 in, 8 out]
                      n506 = for {
                        N: 3 -> [_]
                        shift-right: [w1083] -> w1061
                        shift-left: w1065 -> [w1081]
                        n507 = Search and Replace String(input string=w1081, search string="0", offset=4 ("offset (0)")) -> (result string=w1083:string)  [unwired: 1 in, 7 out]
                      }
                      n508 = Concatenate Strings(w1061, "_" ("replace string (\"\")"), w1063) -> (w1060:string)
                      "date/time string 2" <- w1060
                      n509 = Build Array(w1071, w1072, w1060) -> (w1070:string[])
                      n510 = Build Array(w1071, w1072, w1060, "Calibration_LOG.txt" ("element")) -> (w1074:string[])
                      n511 = Array of Strings to Path(0:w1070) -> (2:w1069:path)  [unwired: 1 out]
                      "Folder" <- w1069
                      n512 = Array of Strings to Path(0:w1074) -> (2:→"calibration log":path)  [unwired: 1 out]
                      n513 = Create Folder(path (use dialog)=w1069) -> ()  [unwired: 2 in, 3 out]
                    }
                    frame #1 {
                      n514 = for {
                        N: 11 -> [_]
                        shift-right: [w1108] -> w1087
                        shift-left: w1089 -> [w1118]
                        shift-right: [w1111] -> w1086
                        shift-left: w1088 -> [w1117]
                        tunnel: w1085 -> [w1104]
                        i -> [w1114]
                        n515 = xnode "Invoke Method"("FPGA VI Reference In"=w1118, "error in"=w1117) -> ("FPGA VI Reference Out"=w1116:refnum<k20>, "error out"=w1115:errorcluster)  [unwired: 1 in]
                        n516 = Increment(x=w1114) -> (x+1=w1113:i32)
                        n517 = Number To Decimal String(number=w1113) -> (decimal integer string=w1112:string)  [unwired: 1 in]
                        n518 = flat-sequence {
                          tunnel: w1116 -> [w1129]
                          tunnel: w1115 -> [w1128]
                          tunnel: w1112 -> [w1127]
                          tunnel: [w1129] -> w1110
                          tunnel: [w1128] -> w1109
                          tunnel: [w1122] -> w1105
                          tunnel: w1104 -> [w1122]
                          tunnel: [w1121] -> w1091
                          tunnel: w1110 -> [w1137]
                          tunnel: w1109 -> [w1136]
                          tunnel: [w1137] -> w1107
                          tunnel: [w1136] -> w1106
                          tunnel: w1105 -> [w1134]
                          tunnel: [w1134] -> w1103
                          tunnel: [w1133] -> w1092
                          tunnel: w1091 -> [w1133]
                          tunnel: w1107 -> [w1177]
                          tunnel: w1106 -> [w1176]
                          tunnel: w1103 -> [w1155]
                          tunnel: [w1175] -> w1102
                          tunnel: [w1174] -> w1101
                          tunnel: [w1148] -> w1100
                          tunnel: [w1147] -> w1099
                          tunnel: [w1146] -> w1098
                          tunnel: [w1145] -> w1097
                          tunnel: w1092 -> [w1138]
                          tunnel: w1102 -> [w1204]
                          tunnel: w1101 -> [w1205]
                          tunnel: w1100 -> [w1201]
                          tunnel: w1099 -> [w1200]
                          tunnel: w1098 -> [w1199]
                          tunnel: w1097 -> [w1198]
                          tunnel: [w1203] -> w1096
                          tunnel: [w1195] -> w1095
                          tunnel: [w1192] -> w1094
                          tunnel: [w1191] -> w1093
                          tunnel: [w1270] -> w1111
                          tunnel: [w1271] -> w1108
                          tunnel: w1096 -> [w1273]
                          tunnel: w1095 -> [w1272]
                          tunnel: w1094 -> [w1268]
                          tunnel: w1093 -> [w1267]
                          frame #0 {
                            w1119 = dbl[] [] ("mean")
                            n519 = local read "Report"() -> (w1124:string)
                            n520 = local write "mean"(w1119) -> ()
                            n521 = local write "median"(w1119) -> ()
                            n522 = local write "max"(w1119) -> ()
                            n523 = local write "min"(w1119) -> ()
                            n524 = local write "Value to compare"(w1119) -> ()
                            n525 = Concatenate Strings("\nAcquiring file: ", w1127, "/11\n" ("string"), w1124) -> (w1123:string)
                            n526 = for {
                              N: 1 -> [_]
                              shift-right: [w1130] -> w1121
                              shift-left: _ -> [w1131]
                              n527 = Add(x=w1131, y=0.001) -> (x+y=w1130:dbl)
                            }
                            n528 = local write "Report"(w1123) -> ()
                          }
                          frame #1 {
                            n529 = Wait (ms)(milliseconds to wait=u32 1000) -> ()  [unwired: 1 out]
                          }
                          frame #2 {
                            n530 = local read "Frecuencia de muestreo y módulo CRIO"() -> (w1173:T3)
                            n531 = local read "Frecuencia de muestreo (Hz)"() -> (w1171:dbl)
                            n532 = Number To Fractional String(number=w1138) -> (F-format string=w1152:string)  [unwired: 3 out]
                            n533 = local read "Escaneos de la FIFO por canal"() -> (w1170:u32)
                            n534 = xnode "Read/Write Control"("FPGA VI Reference In"=w1177, "error in"=w1176, "Fotocélula"=TRUE ("Adquirir")) -> ("FPGA VI Reference Out"=w1181:refnum<k20>, "error out"=w1180:errorcluster)
                            n535 = local read "Nº de acelerómetros"() -> (w1168:i32)
                            n536 = local read "Count(mSec)"() -> (w1172:u32)
                            n537 = local read "Nº inductivos"() -> (w1169:i32)
                            n538 = Search and Replace String(input string=w1152, search string="." ("replace string (\"\")")) -> (result string=w1150:string)  [unwired: 1 in, 8 out]
                            n539 = for {
                              N: 3 -> [_]
                              shift-right: [w1189] -> w1153
                              shift-left: w1150 -> [w1187]
                              n540 = Search and Replace String(input string=w1187, search string="0", offset=4 ("offset (0)")) -> (result string=w1189:string)  [unwired: 1 in, 7 out]
                            }
                            n541 = xnode "Read/Write Control"("FPGA VI Reference In"=w1181, "error in"=w1180, "Data Rate"=w1173, "Digital?"=TRUE, "Count(mSec)"=w1172) -> ("FPGA VI Reference Out"=w1183:refnum<k20>, "error out"=w1182:errorcluster)
                            n542 = Format Date/Time String(time format string (%c)="%Y-%m-%d-%H-%M-%S") -> (date/time string=w1154:string)  [unwired: 2 in]
                            n543 = Add(x=w1169, y=w1168) -> (x+y=w1167:i32)
                            n544 = call "DMACalc.vi"("Number of Channels"=w1167, "Number of Samples"=w1170, "Rate (Hz)"=w1171) -> ("Block Size"=w1147:u32, "Time to Acquire Block (ms)"=w1148:i32, "Host Buffer Size"=w1166:u32)  [unwired: 6 in]
                            n545 = xnode "Invoke Method"("FPGA VI Reference In"=w1183, "error in"=w1182, "Requested Depth"=w1166) -> ("FPGA VI Reference Out"=w1185:refnum<k20>, "error out"=w1184:errorcluster)  [unwired: 1 out]
                            n546 = Concatenate Strings(w1153, "_" ("replace string (\"\")"), w1154, ".bin" ("string")) -> (w1161:string)
                            n547 = Build Array("c", "Calibration" ("element"), w1155, w1161) -> (w1160:string[])
                            n548 = xnode "Invoke Method"("FPGA VI Reference In"=w1185, "error in"=w1184) -> ("FPGA VI Reference Out"=w1175:refnum<k20>, "error out"=w1174:errorcluster)
                            n549 = local read "Report"() -> (w1140:string)
                            n550 = Array of Strings to Path(0:w1160) -> (2:w1141:path)  [unwired: 1 out]
                            n551 = Path To String(path=w1141) -> (string=w1144:string)
                            n552 = Get Date/Time In Seconds() -> (seconds since 1Jan1904=→"Inicio pasada 2":timestamp)
                            n553 = Concatenate Strings("\nFile created: ", w1144, "\n", w1140) -> (w1139:string)
                            n554 = Open/Create/Replace File(file path (use dialog)=w1141, operation (0:open)=T5."replace or create", access (0:read/write)=enum16{"read/write", "read-only", "write-only"}."read/write", disable buffering (F)=TRUE) -> (refnum out=w1146:refnum<file>, error out=w1145:errorcluster)  [unwired: 1 in, 2 out]
                            n555 = local write "Report"(w1139) -> ()
                          }
                          frame #3 {
                            n556 = while "Data Acquisition" {
                              tunnel: w1204 -> [w1230]
                              shift-right: [w1237] -> _
                              shift-left: u32 0 ("t") -> [w1233]
                              tunnel: w1201 -> [w1238]
                              tunnel: w1200 -> [w1236]
                              shift-right: [w1239] -> w1195
                              shift-left: w1205 -> [w1229]
                              tunnel: [w1234] -> w1203
                              tunnel: w1199 -> [w1219]
                              tunnel: [w1220] -> w1192
                              shift-right: [w1218] -> w1191
                              shift-left: w1198 -> [w1227]
                              stop <- w1235 stop-if-true
                              # "Detector de presencia"
                              # "Mide el tiempo de paso del tren y con ello se puede calcular\nla velocidad la unidad"
                              n557 = xnode "Invoke Method"("FPGA VI Reference In"=w1230, "error in"=w1229, "Number of Elements"=w1233, "Timeout (ms)"=0) -> ("FPGA VI Reference Out"=w1217:refnum<k20>, "error out"=w1216:errorcluster, "Data"=w1228:fxp<+/-,24,4>[], "Elements Remaining"=w1231:u32)
                              n558 = case "Data Ready" shown="Default" w1233 {
                                tunnel: w1238 -> [w1244 _]
                                tunnel: [w1243 u32 0 ("t")] -> w1237
                                tunnel: w1236 -> [w1245 _]
                                tunnel: w1231 -> [w1242 _]
                                tunnel: w1228 -> [_ w1255]
                                tunnel: w1227 -> [w1241 w1257]
                                tunnel: [w1241 w1256] -> w1218
                                tunnel: w1219 -> [w1240 w1254]
                                tunnel: [w1240 w1253] -> w1220
                                frame 0 {
                                n559 = Greater Or Equal?(x=w1242, y=w1245) -> (x >= y?=w1246:bool)
                                n560 = case shown="False" w1246 {
                                tunnel: [u32 0 ("Block Size") w1250] -> w1243
                                tunnel: [w1249 0 ("t")] -> w1247
                                tunnel: w1244 -> [w1249 _]
                                tunnel: w1245 -> [_ w1250]
                                frame False {
                                }
                                frame True {
                                }
                                }
                                n561 = call "WaitMinTimeBetweenCall.vi"("Minimum ms between calls"=w1247) -> ()  [unwired: 2 in]
                                }
                                frame Default {
                                n562 = To Single Precision Float(number=w1255) -> (single precision float=w1252:sgl[])
                                n563 = Write to Binary File(file (use dialog)=w1254, data=w1252, error in=w1257, 5:FALSE ("prepend array or string size? (T)"), 9:T6."little-endian" ("byte order (0:big-endian, network order)")) -> (refnum out=w1253:refnum<file>, error out=w1256:errorcluster)  [unwired: 2 out]
                                }
                              }
                              n564 = local read "Inicio pasada 2"() -> (w1208:timestamp)
                              n565 = Get Date/Time In Seconds() -> (seconds since 1Jan1904=w1209:timestamp)
                              n566 = xnode ("CheckLate")("FPGA VI Reference In"=w1217, "error in"=w1216) -> ("FPGA VI Reference Out"=w1211:refnum<k20>, "error out"=w1225:errorcluster, "Buffer Underflow"=w1206:bool, "Buffer Overflow"=w1207:bool)
                              n567 = To Double Precision Float(number=w1209) -> (double precision float=w1214:dbl)
                              n568 = To Double Precision Float(number=w1208) -> (double precision float=w1215:dbl)
                              n569 = Subtract(x=w1214, y=w1215) -> (x-y=w1222:dbl)
                              "Acquiring time" <- w1222
                              n570 = local write "Buffer Overflow"(w1207) -> ()
                              n571 = local write "Buffer Underflow"(w1206) -> ()
                              n572 = Greater?(x=w1222, y=1.0 ("Tiempo de adquisición")) -> (0:w1213:bool)
                              n573 = call "ErrorOverFlow.vi"("Buffer Overflow"=w1207) -> ("error out"=w1223:errorcluster)
                              n574 = call "ErrorUnderFlow.vi"("Buffer Overflow"=w1206) -> ("error out"=w1224:errorcluster)
                              n575 = Merge Errors(w1225, w1224, w1223) -> (w1212:errorcluster)
                              n576 = Unbundle By Name(w1218) -> ("status"=w1221:bool)
                              n577 = Unbundle By Name(w1212) -> ("status"=w1226:bool)
                              n578 = Compound Arithmetic op=OR(w1226, w1213, w1221) -> (w1235:bool)
                              n579 = case "Flush" shown="True" w1235 {
                                tunnel: w1211 -> [w1261 w1266]
                                tunnel: w1212 -> [w1262 w1265]
                                tunnel: [w1262 w1264] -> w1239
                                tunnel: [w1261 w1263] -> w1234
                                frame False {
                                }
                                frame True {
                                n580 = xnode "Invoke Method"("FPGA VI Reference In"=w1266, "error in"=w1265) -> ("FPGA VI Reference Out"=w1263:refnum<k20>, "error out"=w1264:errorcluster)
                                }
                              }
                            }
                            n581 = call "Reporting_error.vi"("error out 2"=w1195, "Concept"="FPGA ") -> ("Reporting"=w1197:string)  [unwired: 1 in]
                            n582 = local read "Report"() -> (w1194:string)
                            n583 = Concatenate Strings(w1197, w1194) -> (w1196:string)
                            n584 = local write "Report"(w1196) -> ()
                          }
                          frame #4 {
                            n585 = xnode "Read/Write Control"("FPGA VI Reference In"=w1273, "error in"=w1272, "Stop"=TRUE) -> ("FPGA VI Reference Out"=w1274:refnum<k20>, "error out"=w1275:errorcluster)
                            n586 = Close File(refnum=w1268, error in=w1267) -> ()  [unwired: 2 out]
                            n587 = xnode "Invoke Method"("FPGA VI Reference In"=w1274, "error in"=w1275) -> ("FPGA VI Reference Out"=w1271:refnum<k20>, "error out"=w1270:errorcluster)
                          }
                        }
                      }
                    }
                  }
                }
                frame "Acel_calib" {
                  n588 = local read "Folder"() -> (w1286:path)
                  n589 = local read "Frecuencia de muestreo (Hz)"() -> (w1292:dbl)
                  n590 = local read "Nº de acelerómetros"() -> (w1287:i32)
                  n591 = local read "Nº inductivos"() -> (w1288:i32)
                  n592 = local read "Pattern frequency (Hz)"() -> (w1293:dbl)
                  n593 = call <vilib>:"Recursive File List.vi"("Folder Path"=w1286) -> ("All Files in Dir"=w1291:path[])  [unwired: 6 in, 4 out]
                  n594 = Array Size(array=w1291) -> (size(s)=→"Nº meas":i32)
                  n595 = Add(x=w1288, y=w1287) -> (x+y=w1290:i32)
                  n596 = flat-sequence {
                    tunnel: w1291 -> [w1303]
                    tunnel: [w1303] -> w1299
                    tunnel: [w1302] -> w1298
                    tunnel: w1290 -> [w1302]
                    tunnel: [w1301] -> w1297
                    tunnel: w1292 -> [w1301]
                    tunnel: [w1300] -> w1296
                    tunnel: w1293 -> [w1300]
                    tunnel: [w1310] -> w1295
                    tunnel: [w1309] -> w1294
                    tunnel: w1299 -> [w1311]
                    tunnel: w1298 -> [w1308]
                    tunnel: w1297 -> [w1307]
                    tunnel: w1296 -> [w1306]
                    tunnel: [w1305] -> w1276
                    tunnel: w1295 -> [w1423]
                    tunnel: w1294 -> [w1412]
                    tunnel: [w1404] -> w1280
                    tunnel: [TRUE] -> w1279
                    tunnel: [w1438] -> w1277
                    tunnel: [w1413] -> w1278
                    tunnel: w1276 -> [w1408]
                    frame #0 {
                      "Valid\nindex" <- i32[] []
                    }
                    frame #1 {
                      n597 = for {
                        tunnel: w1311 -> [w1333] mode=indexing
                        tunnel: [w1323] -> w1310 mode=indexing
                        tunnel: [w1313] -> w1309 mode=indexing
                        tunnel: w1308 -> [w1321]
                        tunnel: w1307 -> [w1320]
                        tunnel: w1306 -> [w1319]
                        tunnel: [w1312] -> w1305 mode=indexing
                        n598 = Read from Binary File(5:sgl 1.25, 9:T6."little-endian" ("byte order (0:big-endian, network order)"), 10:-1 ("count (1)"), 11:w1333) -> (2:w1334:sgl[])  [unwired: 1 in, 4 out]
                        n599 = case shown="10" w1321 {
                          tunnel: [w1351 w1364 w1374] -> w1313
                          tunnel: w1334 -> [w1352 w1362 w1375]
                          frame 9, Default {
                            n600 = Decimate 1D Array(w1352) -> (w1353:sgl[], w1361:sgl[], w1360:sgl[], w1356:sgl[], w1355:sgl[], w1357:sgl[], w1358:sgl[], w1359:sgl[], w1354:sgl[])
                            n601 = Build Array(w1353, w1361, w1360, w1356, w1355, w1357, w1358, w1359, w1354) -> (w1351:sgl[][])
                          }
                          frame 10 {
                            n602 = Decimate 1D Array(w1362) -> (w1363:sgl[], w1373:sgl[], w1372:sgl[], w1368:sgl[], w1367:sgl[], w1369:sgl[], w1370:sgl[], w1371:sgl[], w1366:sgl[], w1365:sgl[])
                            n603 = Build Array(w1363, w1373, w1372, w1368, w1367, w1369, w1370, w1371, w1366, w1365) -> (w1364:sgl[][])
                          }
                          frame 5 {
                            n604 = Decimate 1D Array(w1375) -> (w1376:sgl[], w1380:sgl[], w1379:sgl[], w1378:sgl[], w1377:sgl[])
                            n605 = Build Array(w1376, w1380, w1379, w1378, w1377) -> (w1374:sgl[][])
                          }
                        }
                        n606 = for {
                          tunnel: w1313 -> [w1383] mode=indexing
                          tunnel: [w1386] -> w1330 mode=indexing
                          tunnel: w1320 -> [w1385]
                          tunnel: w1319 -> [w1384]
                          n607 = call-poly <vilib>:"Basic Averaged DC-RMS.vi"("signal in"=w1383) -> ("DC value"=w1396:dbl)  [unwired: 7 in, 3 out]
                          n608 = Array Size(array=w1383) -> (size(s)=→"size(s) 3":i32)
                          n609 = Subtract(x=w1383, y=w1396) -> (x-y=w1392:dbl[])
                          n610 = Divide(x=w1385, y=w1384) -> (x/y=w1393:dbl)
                          n611 = Array Size(array=w1392) -> (size(s)=w1394:i32)
                          n612 = Subtract(x=w1394, y=w1393) -> (x-y=w1395:dbl)
                          n613 = for {
                            N: w1395 -> [_]
                            tunnel: w1393 -> [w1398]
                            tunnel: [w1401] -> w1381 mode=indexing
                            tunnel: w1392 -> [w1400]
                            i -> [w1399]
                            n614 = Array Subset(array=w1400, index=w1399, length=w1398) -> (w1397:dbl[])
                            n615 = call-poly <vilib>:"RMS.vi"("X"=w1397) -> ("rms value"=w1401:dbl)  [unwired: 1 out]
                          }
                          n616 = Greater?(x=w1381, y=0.004 ("threshold y")) -> (0:w1390:bool[])
                          n617 = Search 1D Array(1D array=w1390, element=TRUE) -> (index of element=w1388:i32)  [unwired: 1 in]
                          n618 = Not Equal?(x=w1388, y=-1) -> (x != y?=w1386:bool)
                        }
                        n619 = Array Size(array=w1313) -> (size(s)=→"size(s)":i32[])
                        n620 = while {
                          tunnel: w1330 -> [w1350]
                          shift-right: [w1342] -> _
                          shift-left: 0 ("index of element") -> [w1347]
                          shift-right: [w1343] -> w1322
                          shift-left: 0 ("index of element") -> [w1344]
                          tunnel: [w1341] -> w1318 mode=indexing
                          i -> [w1345]
                          stop <- w1348 stop-if-true
                          n621 = Add(x=w1344, y=w1345) -> (x+y=w1343:i32)
                          n622 = Search 1D Array(1D array=w1350, element=TRUE, start index (0)=w1347) -> (index of element=w1341:i32)
                          n623 = Equal?(x=w1341, y=-1) -> (x = y?=w1348:bool)
                          n624 = Increment(x=w1341) -> (x+1=w1342:i32)
                        }
                        n625 = Delete From Array(array=w1318, length=1) -> (array with subset deleted=w1317:i32[])  [unwired: 1 in, 1 out]
                        n626 = Array Size(array=w1317) -> (size(s)=w1326:i32)
                        n627 = Equal?(x=w1322, y=1) -> (x = y?=w1325:bool)
                        n628 = Equal?(x=w1326, y=1) -> (x = y?=w1324:bool)
                        n629 = And(x=w1324, y=w1325) -> (x .and. y?=w1323:bool)
                        n630 = case shown="True" w1323 {
                          tunnel: w1317 -> [_ w1340]
                          frame False {
                          }
                          frame True {
                            n631 = local read "Valid\nindex"() -> (w1338:i32[])
                            n632 = Insert Into Array(array=w1338, new element=w1340) -> (w1339:i32[])  [unwired: 1 in]
                            n633 = local write "Valid\nindex"(w1339) -> ()
                          }
                        }
                        n634 = Array Size(array=w1313) -> (size(s)=w1315:i32[])
                        n635 = Index Array(array=w1315, index=1) -> (element=w1312:i32)
                      }
                    }
                    frame #2 {
                      w1422 = 0 ("index of element")
                      (unwired) 0 ("index of element")
                      n636 = local read "Valid\nindex"() -> (w1428:i32[])
                      n637 = Array Max & Min(array=w1408) -> (min value=w1405:i32)  [unwired: 3 out]
                      n638 = Sort 1D Array(array=w1428) -> (sorted array=w1424:i32[])
                      "sorted array" <- w1424
                      n639 = Decrement(x="Accelerometer") -> (x-1=w1403:i32)
                      n640 = for {
                        tunnel: w1424 -> [w1459] mode=indexing
                        shift-right: [w1459] -> _
                        shift-left: -1 ("y") -> [w1460]
                        tunnel: [w1459] -> w1433 mode=indexing if=w1458
                        shift-right: [w1455] -> _
                        shift-left: 0 ("y") -> [w1456]
                        tunnel: [w1455] -> w1431 mode=indexing
                        n641 = Not Equal?(x=w1459, y=w1460) -> (x != y?=w1458:bool)
                        n642 = Increment(x=w1456) -> (x+1=w1457:i32)
                        n643 = Select(t=1 ("y"), s=w1458, f=w1457) -> (s? t:f=w1455:i32)
                      }
                      "Array" <- w1433
                      "Array 3" <- w1431
                      n644 = Delete From Array(array=w1412, index (dim 1)=w1403) -> (deleted portion=w1406:sgl[][])  [unwired: 3 in, 1 out]
                      n645 = for {
                        tunnel: w1423 -> [w1465] mode=indexing
                        shift-right: [w1464] -> _
                        shift-left: w1412 -> [w1466]
                        shift-right: [w1461] -> _
                        shift-left: 0 ("index of element") -> [w1462]
                        i -> [w1463]
                        n646 = case shown="False" w1465 {
                          tunnel: w1466 -> [w1472 w1474]
                          tunnel: [w1471 w1474] -> w1464
                          tunnel: w1463 -> [w1470 _]
                          tunnel: w1462 -> [w1467 w1473]
                          tunnel: [w1468 w1473] -> w1461
                          frame False {
                            n647 = Subtract(x=w1470, y=w1467) -> (x-y=w1469:i32)
                            n648 = Delete From Array(array=w1472, index (dim 0)=w1469) -> (array with subset deleted=w1471:sgl[][][])  [unwired: 3 in, 1 out]
                            n649 = Increment(x=w1467) -> (x+1=w1468:i32)
                          }
                          frame True {
                          }
                        }
                      }
                      n650 = Array Subset(array=w1406, index (col)=0 ("index"), length (col)=w1405) -> (w1404:sgl[][])  [unwired: 2 in]
                      n651 = Array Max & Min(array=w1431) -> (max value=→"max value":i32, max index (indices)=w1429:i32)  [unwired: 2 out]
                      "max index(es)" <- w1429
                      n652 = Index Array(array=w1424, index=w1429) -> (element=w1413:i32)
                      "element" <- w1413
                      n653 = local read "Frecuencia de muestreo (Hz)"() -> (w1411:dbl)
                      n654 = Equal?(x=w1428, y=w1413) -> (x = y?=w1426:bool[])
                      n655 = Boolean To (0,1)(Boolean=w1426) -> (0, 1=w1425:i16[])
                      n656 = Add Array Elements(numeric array=w1425) -> (sum=w1417:i16)
                      n657 = Equal?(x=w1413, y=w1422) -> (x = y?=w1420:bool)
                      n658 = Equal?(x=w1422, y=w1417) -> (x = y?=w1419:bool)
                      n659 = Increment(x=w1413) -> (x+1=w1427:i32)
                      n660 = local read "Nº meas"() -> (w1439:i32)
                      n661 = Not And(1:w1419, 2:w1420) -> (0:w1418:bool)
                      n662 = for {
                        tunnel: w1404 -> [w1453] mode=indexing
                        tunnel: w1411 -> [w1451]
                        tunnel: [w1450] -> w1410 mode=indexing
                        n663 = Reciprocal(x=w1451) -> (1/x=w1452:dbl)
                        n664 = Bundle By Name("Y"=w1453, "dt"=w1452) -> (w1450:waveform(sgl))  [unwired: 1 in]
                      }
                      n665 = Number To Decimal String(number=w1427) -> (decimal integer string=w1415:string)  [unwired: 1 in]
                      n666 = Select(t=w1415, s=w1418, f=" NONE ") -> (s? t:f=w1416:string)
                      n667 = Number To Decimal String(number=w1417) -> (decimal integer string=w1445:string)  [unwired: 1 in]
                      n668 = Number To Decimal String(number=w1439) -> (decimal integer string=w1443:string)  [unwired: 1 in]
                      n669 = Divide(x=w1417, y=w1439) -> (x/y=w1441:dbl)
                      n670 = for {
                        tunnel: w1410 -> [w1449] mode=indexing
                        tunnel: [w1446] -> w1409 mode=concatenating
                        n671 = call "Convert to Dynamic Data"("Waveform"=w1449) -> ("Dynamic Data Type"=w1448:dynamicdata)  [unwired: 3 in]
                        n672 = call "Tone Measurements"("Signals"=w1448) -> ("Frequency"=w1447:dynamicdata)  [unwired: 9 in, 1 out]
                        n673 = call "Convert from Dynamic Data"("Dynamic Data Type"=w1447) -> ("Array"=w1446:dbl[])  [unwired: 3 in]
                      }
                      "Frequency" <- w1409
                      n674 = Greater?(x=w1441, y=0.6) -> ()  [unwired: 1 out]
                      n675 = Concatenate Strings("\nACCELEROMETER DETECTOR:\n\nAccelerometer detected: ", w1416, " \nAccelerometer detected in  ", w1445, " of ", w1443, " measurements\n------------------------------------------------------------------------------------------------------------------------------------------------") -> (w1438:string)
                    }
                  }
                  n676 = local read "Report"() -> (w1281:string)
                  n677 = Concatenate Strings(w1277, w1281) -> (w1282:string)
                  n678 = local write "Report"(w1282) -> ()
                  "Accel.detected" <- w1278
                }
                frame "Acel_frequency" {
                  n679 = local read "Low cutoff freq"() -> (w1479:dbl)
                  n680 = local read "Frequency"() -> (w1480:dbl[])
                  n681 = local read "Frecuencia de muestreo (Hz)"() -> (w1482:dbl)
                  n682 = for {
                    tunnel: w1477 -> [w1513] mode=indexing
                    tunnel: w1482 -> [w1511]
                    tunnel: [w1510] -> w1481 mode=indexing
                    n683 = Reciprocal(x=w1511) -> (1/x=w1512:dbl)
                    n684 = Bundle By Name("Y"=w1513, "dt"=w1512) -> (w1510:waveform(sgl))  [unwired: 1 in]
                  }
                  "Waveform Graph" <- w1481
                  n685 = local read "Pattern frequency (Hz)"() -> (w1483:dbl)
                  n686 = Less?(x=w1480, y=w1479) -> (x < y?=w1475:bool[])
                  n687 = for {
                    tunnel: w1475 -> [w1500] mode=indexing
                    shift-right: [w1499] -> w1476
                    shift-left: w1477 -> [w1501]
                    shift-right: [w1496] -> _
                    shift-left: 0 ("index of element") -> [w1497]
                    i -> [w1498]
                    n688 = case shown="False" w1500 {
                      tunnel: w1501 -> [w1507 w1509]
                      tunnel: [w1506 w1509] -> w1499
                      tunnel: w1498 -> [w1505 _]
                      tunnel: w1497 -> [w1502 w1508]
                      tunnel: [w1503 w1508] -> w1496
                      frame False {
                        n689 = Subtract(x=w1505, y=w1502) -> (x-y=w1504:i32)
                        n690 = Delete From Array(array=w1507, index (row)=w1504) -> (array with subset deleted=w1506:sgl[][])  [unwired: 2 in, 1 out]
                        n691 = Increment(x=w1502) -> (x+1=w1503:i32)
                      }
                      frame True {
                      }
                    }
                  }
                  n692 = flat-sequence {
                    tunnel: w1476 -> [w1520]
                    tunnel: w1482 -> [w1517]
                    tunnel: w1483 -> [w1514]
                    tunnel: [w1522] -> w1495
                    tunnel: [w1516] -> w1494
                    tunnel: [w1515] -> w1493
                    tunnel: [w1514] -> w1492
                    tunnel: w1495 -> [w1599]
                    tunnel: w1494 -> [w1581]
                    tunnel: w1493 -> [w1598]
                    tunnel: w1492 -> [w1597]
                    tunnel: [w1599] -> w1487
                    tunnel: [w1583] -> w1484
                    tunnel: [w1582] -> w1486
                    tunnel: [w1581] -> _
                    frame #0 {
                      n693 = for {
                        tunnel: w1520 -> [w1572] mode=indexing
                        tunnel: w1517 -> [w1571]
                        tunnel: w1514 -> [w1567]
                        tunnel: [w1548] -> w1516 mode=indexing
                        tunnel: [w1542] -> w1515 mode=indexing
                        n694 = Reciprocal(x=w1571) -> (1/x=w1573:dbl)
                        n695 = Bundle By Name("Y"=w1572, "dt"=w1573) -> (w1570:waveform(sgl))  [unwired: 1 in]
                        n696 = call-poly <vilib>:"FFT Spectrum (Mag-Phase).vi"("time signal"=w1570) -> ("magnitude"=w1569:cluster{"f0":dbl, "df":dbl, "magnitude":dbl[]})  [unwired: 6 in, 4 out]
                        n697 = Unbundle By Name(w1569) -> ("magnitude"=w1561:dbl[], "df"=w1543:dbl)
                        n698 = Multiply(x=1.03, y=w1567) -> (x*y=w1564:dbl)
                        n699 = Multiply(x=w1567, y=0.97 ("x")) -> (x*y=w1565:dbl)
                        n700 = Divide(x=w1565, y=w1543) -> (x/y=w1562:dbl)
                        n701 = Divide(x=w1564, y=w1543) -> (x/y=w1559:dbl)
                        n702 = Array Max & Min(array=w1561) -> (max value=w1554:dbl, max index (indices)=w1544:i32)  [unwired: 2 out]
                        n703 = Array Size(array=w1561) -> (size(s)=w1560:i32)
                        n704 = Multiply(x=w1544, y=w1543) -> (x*y=w1542:dbl)
                        n705 = Subtract(x=w1560, y=w1559) -> (x-y=w1558:dbl)
                        n706 = In Range and Coerce(upper limit=w1564, x=w1542, lower limit=w1565) -> (In Range?=w1547:bool)  [unwired: 1 out]
                        n707 = Array Subset(array=w1561, index=w1559, length=w1558) -> (w1557:dbl[])
                        n708 = Array Subset(array=w1561, index=0, length=w1562) -> (w1556:dbl[])
                        n709 = Array Max & Min(array=w1557) -> (max value=w1555:dbl)  [unwired: 3 out]
                        n710 = Array Max & Min(array=w1556) -> (max value=w1553:dbl)  [unwired: 3 out]
                        n711 = Divide(x=w1554, y=w1553) -> (x/y=w1551:dbl)
                        n712 = Divide(x=w1554, y=w1555) -> (x/y=w1552:dbl)
                        n713 = Greater?(x=w1552, y=3.0) -> (0:w1546:bool)
                        n714 = Greater?(x=w1551, y=3.0) -> (0:w1545:bool)
                        n715 = Compound Arithmetic op=AND(w1547, w1546, w1545) -> (w1548:bool)
                      }
                      n716 = for {
                        shift-right: [w1529] -> w1522
                        shift-left: w1520 -> [w1530]
                        tunnel: w1516 -> [w1528] mode=indexing
                        shift-right: [w1525] -> _
                        shift-left: 0 ("index of element") -> [w1526]
                        shift-right: [w1523] -> w1519
                        shift-left: w1515 -> [w1524]
                        i -> [w1527]
                        n717 = case shown="True" w1528 {
                          tunnel: w1530 -> [w1538 w1541]
                          tunnel: [w1537 w1541] -> w1529
                          tunnel: w1527 -> [w1536 _]
                          tunnel: w1526 -> [w1535 w1540]
                          tunnel: [w1534 w1540] -> w1525
                          tunnel: w1524 -> [w1533 w1539]
                          tunnel: [w1531 w1539] -> w1523
                          frame False {
                            n718 = Subtract(x=w1536, y=w1535) -> (x-y=w1532:i32)
                            n719 = Delete From Array(array=w1538, index (row)=w1532) -> (array with subset deleted=w1537:sgl[][])  [unwired: 2 in, 1 out]
                            n720 = Increment(x=w1535) -> (x+1=w1534:i32)
                            n721 = Delete From Array(array=w1533, index=w1532) -> (array with subset deleted=w1531:dbl[])  [unwired: 1 in, 1 out]
                          }
                          frame True {
                          }
                        }
                      }
                      n722 = call <vilib>:"Std Deviation and Variance.vi"("X"=w1519) -> ("mean"=→"Mean\nfrequency":dbl)  [unwired: 1 in, 2 out]
                    }
                    frame #1 {
                      w1578 = "\r"
                      n723 = for {
                        tunnel: w1581 -> [w1607] mode=indexing
                        tunnel: w1598 -> [w1626] mode=indexing
                        tunnel: w1597 -> [w1625]
                        tunnel: [w1608] -> w1595 mode=indexing
                        shift-right: [w1602] -> w1593
                        shift-left: 0 -> [w1603]
                        i -> [w1628]
                        n724 = Increment(x=w1628) -> (x+1=w1627:i32)
                        n725 = Select(t=1, s=w1607, f=0) -> (s? t:f=w1604:i32)
                        n726 = Divide(x=w1626, y=w1625) -> (x/y=w1623:dbl)
                        n727 = Select(t="TRUE", s=w1607, f="FALSE") -> (s? t:f=w1617:string)
                        n728 = Number To Decimal String(number=w1627) -> (decimal integer string=w1620:string)  [unwired: 1 in]
                        n729 = Number To Fractional String(number=w1626, precision (6)=i16 2) -> (F-format string=w1614:string)  [unwired: 2 in]
                        n730 = Add(x=w1604, y=w1603) -> (x+y=w1602:i32)
                        n731 = Greater Than 0?(x=w1623) -> (x > 0?=w1624:bool)
                        n732 = case shown="True" w1624 {
                          tunnel: w1623 -> [w1636 w1638]
                          tunnel: [w1632 w1640] -> w1622
                          tunnel: ["-" " "] -> w1612
                          frame False {
                            n733 = Subtract(x=1.0, y=w1636) -> (x-y=w1634:dbl)
                            n734 = Multiply(x=100.0, y=w1634) -> (x*y=w1632:dbl)
                          }
                          frame True {
                            n735 = Decrement(x=w1638) -> (x-1=w1639:dbl)
                            n736 = Multiply(x=100.0, y=w1639) -> (x*y=w1640:dbl)
                          }
                        }
                        n737 = Number To Fractional String(number=w1622, precision (6)=i16 2) -> (F-format string=w1611:string)  [unwired: 2 in]
                        n738 = Concatenate Strings("\n\nMeasurement: ", w1620, "\r", "Frequency valid: ", w1617, "\r", "Frequency: ", w1614, ", ", w1612, w1611, " % of error in frequency", "\r") -> (w1608:string)
                      }
                      n739 = Array Size(array=w1581) -> (size(s)=w1592:i32)
                      n740 = Number To Decimal String(number=w1592) -> (decimal integer string=w1587:string)  [unwired: 1 in]
                      n741 = Number To Decimal String(number=w1593) -> (decimal integer string=w1579:string)  [unwired: 1 in]
                      n742 = Divide(x=w1593, y=w1592) -> (x/y=w1576:dbl)
                      n743 = Greater?(x=w1576, y=0.8) -> (0:w1582:bool)
                      n744 = Multiply(x=100.0, y=w1576) -> (x*y=w1575:dbl)
                      n745 = Number To Fractional String(number=w1575, precision (6)=i16 2) -> (F-format string=w1586:string)  [unwired: 2 in]
                      n746 = Select(t="OK\n------------------------------------------------------------------------", s=w1582, f="FAIL (REPEAT ACEL CALIBRATION)\n------------------------------------------------------------------------") -> (s? t:f=w1584:string)
                      n747 = Concatenate Strings("FREQUENCY TEST:\n \n- MEASUREMENT OK IF +/- 5% FREQ PATTERN\n\n- FREQUENCY ANALYSYS MORE THAN 80% OF THE MEASUREMENTS INSIDE OF THE RANGE\n", w1595, w1578, w1578, w1579, " measurements OK of ", w1587, " , ", w1586, " %\n\nFREQUENCY ANALYSIS: ", w1584) -> (w1583:string)
                    }
                  }
                  n748 = local read "Report"() -> (w1491:string)
                  n749 = Concatenate Strings(w1484, w1491) -> (w1490:string)
                  n750 = local write "Report"(w1490) -> ()
                }
                frame "Acel_noise" {
                  n751 = local read "Frecuencia de muestreo (Hz)"() -> (w1645:dbl)
                  n752 = local read "Pattern frequency (Hz)"() -> (w1644:dbl)
                  n753 = flat-sequence {
                    tunnel: w1652 -> [w1663]
                    tunnel: [w1679] -> w1649
                    tunnel: w1645 -> [w1678]
                    tunnel: w1644 -> [w1677]
                    tunnel: [w1666] -> w1642
                    tunnel: [w1665] -> w1646
                    frame #0 {
                      n754 = for {
                        tunnel: w1663 -> [w1727] mode=indexing
                        tunnel: [w1720] -> w1683 mode=indexing
                        tunnel: w1678 -> [w1715]
                        tunnel: w1677 -> [w1716]
                        n755 = call-poly <vilib>:"Basic Averaged DC-RMS.vi"("signal in"=w1727) -> ("DC value"=w1728:dbl)  [unwired: 7 in, 3 out]
                        n756 = Subtract(x=w1727, y=w1728) -> (x-y=w1717:dbl[])
                        n757 = Divide(x=w1715, y=w1716) -> (x/y=w1724:dbl)
                        n758 = Array Size(array=w1717) -> (size(s)=w1725:i32)
                        n759 = Subtract(x=w1725, y=w1724) -> (x-y=w1726:dbl)
                        n760 = for {
                          N: w1726 -> [_]
                          tunnel: w1724 -> [w1730]
                          tunnel: [w1733] -> w1718 mode=indexing
                          tunnel: w1717 -> [w1732]
                          i -> [w1731]
                          n761 = Array Subset(array=w1732, index=w1731, length=w1730) -> (w1729:dbl[])
                          n762 = call-poly <vilib>:"RMS.vi"("X"=w1729) -> ("rms value"=w1733:dbl)  [unwired: 1 out]
                        }
                        n763 = Array Max & Min(array=w1718) -> (max value=w1722:dbl, min value=w1721:dbl)  [unwired: 2 out]
                        n764 = call <vilib>:"Std Deviation and Variance.vi"("X"=w1718) -> ("mean"=w1719:dbl)  [unwired: 1 in, 2 out]
                        n765 = call <vilib>:"Median.vi"("X"=w1718) -> ("median"=w1723:dbl)  [unwired: 1 out]
                        n766 = Build Array(w1719, w1723, w1722, w1721) -> (w1720:dbl[])
                      }
                      n767 = Multiply(x=w1683, y=1000 ("median")) -> (x*y=w1662:dbl[][])
                      n768 = Index Array(array=w1662, index (col) #1=0 ("disabled index (col)"), index (col) #2=1 ("index (col)"), index (col) #3=2 ("index (col)"), index (col) #4=3 ("index (col)")) -> (element #1=→"mean":dbl[], element #2=→"median":dbl[], element #3=→"max":dbl[], element #4=→"min":dbl[])  [unwired: 4 in]
                      n769 = for {
                        tunnel: w1662 -> [w1710] mode=indexing
                        tunnel: [w1707] -> w1664 mode=indexing
                        tunnel: [w1705] -> w1653 mode=indexing
                        (unwired) 0.2 ("x")
                        n770 = local read "noise_range"() -> (w1706:dbl)
                        n771 = call <vilib>:"Median.vi"("X"=w1710) -> ("median"=w1705:dbl)  [unwired: 1 out]
                        n772 = Subtract(x=w1705, y=w1706) -> (x-y=w1708:dbl)
                        n773 = Add(x=w1706, y=w1705) -> (x+y=w1709:dbl)
                        n774 = for {
                          tunnel: w1710 -> [w1714] mode=indexing
                          tunnel: w1709 -> [w1713]
                          tunnel: w1708 -> [w1712]
                          tunnel: [w1711] -> w1707 mode=indexing
                          n775 = In Range and Coerce(upper limit=w1713, x=w1714, lower limit=w1712) -> (In Range?=w1711:bool)  [unwired: 1 out]
                        }
                      }
                      "Value to compare" <- w1653
                      n776 = for {
                        tunnel: w1664 -> [w1704] mode=indexing
                        tunnel: [w1703] -> w1680 mode=indexing
                        n777 = And Array Elements(Boolean array=w1704) -> (logical AND=w1703:bool)
                      }
                      n778 = for {
                        shift-right: [w1690] -> w1679
                        shift-left: w1663 -> [w1691]
                        tunnel: w1680 -> [w1689] mode=indexing
                        shift-right: [w1686] -> w1676
                        shift-left: 0 ("index of element") -> [w1687]
                        shift-right: [w1684] -> w1671
                        shift-left: 0 ("index of element") -> [w1685]
                        i -> [w1688]
                        n779 = case shown="False" w1689 {
                          tunnel: w1691 -> [w1698 w1702]
                          tunnel: [w1697 w1702] -> w1690
                          tunnel: w1688 -> [w1696 _]
                          tunnel: w1687 -> [w1695 w1701]
                          tunnel: [w1694 w1701] -> w1686
                          tunnel: w1685 -> [w1692 w1700]
                          tunnel: [w1692 w1699] -> w1684
                          frame False {
                            n780 = Subtract(x=w1696, y=w1695) -> (x-y=w1693:i32)
                            n781 = Delete From Array(array=w1698, index (row)=w1693) -> (array with subset deleted=w1697:sgl[][])  [unwired: 2 in, 1 out]
                            n782 = Increment(x=w1695) -> (x+1=w1694:i32)
                          }
                          frame True {
                            n783 = Increment(x=w1700) -> (x+1=w1699:i32)
                          }
                        }
                      }
                      n784 = Number To Decimal String(number=w1676) -> (decimal integer string=w1674:string)  [unwired: 1 in]
                      n785 = Greater?(x=w1671, y=3) -> (0:w1665:bool)
                      n786 = Select(t="------------------------------------------------------------------------", s=w1665, f="There are not enough correct measurements to calibrate\n\nREPEAT THE ACCELEROMETER CALIBRATION\n------------------------------------------------------------------------") -> (s? t:f=w1667:string)
                      n787 = Concatenate Strings("SIGNAL NOISE ANALYSIS:\n\nFiles erasing by  noise: ", w1674, "\r", w1667) -> (w1666:string)
                    }
                  }
                  n788 = local read "Report"() -> (w1647:string)
                  n789 = Concatenate Strings(w1642, w1647) -> (w1648:string)
                  n790 = local write "Report"(w1648) -> ()
                }
                frame "Acel_result" {
                  n791 = local read "Frecuencia de muestreo (Hz)"() -> (w1745:dbl)
                  n792 = local read "Pattern frequency (Hz)"() -> (w1744:dbl)
                  n793 = local read "Pattern amplitude (g)"() -> (w1743:dbl)
                  n794 = flat-sequence {
                    tunnel: w1746 -> [w1764]
                    tunnel: w1745 -> [w1762]
                    tunnel: w1744 -> [w1761]
                    tunnel: w1743 -> [w1760]
                    tunnel: [w1759] -> w1739
                    tunnel: [w1750] -> _
                    tunnel: [w1749] -> w1734
                    frame #0 {
                      n795 = for {
                        tunnel: w1764 -> [w1778] mode=indexing
                        tunnel: w1762 -> [w1774]
                        tunnel: w1761 -> [w1771]
                        tunnel: [w1772] -> w1769 mode=indexing
                        n796 = call-poly <vilib>:"Basic Averaged DC-RMS.vi"("signal in"=w1778) -> ("DC value"=w1779:dbl)  [unwired: 7 in, 3 out]
                        n797 = Subtract(x=w1778, y=w1779) -> (x-y=w1770:dbl[])
                        n798 = Divide(x=w1774, y=w1771) -> (x/y=w1775:dbl)
                        n799 = Array Size(array=w1770) -> (size(s)=w1776:i32)
                        n800 = Subtract(x=w1776, y=w1775) -> (x-y=w1777:dbl)
                        n801 = for {
                          N: w1777 -> [_]
                          tunnel: w1775 -> [w1781]
                          tunnel: [w1784] -> w1773 mode=indexing
                          tunnel: w1770 -> [w1783]
                          i -> [w1782]
                          n802 = Array Subset(array=w1783, index=w1782, length=w1781) -> (w1780:dbl[])
                          n803 = call-poly <vilib>:"RMS.vi"("X"=w1780) -> ("rms value"=w1784:dbl)  [unwired: 1 out]
                        }
                        n804 = call <vilib>:"Std Deviation and Variance.vi"("X"=w1773) -> ("mean"=w1772:dbl)  [unwired: 1 in, 2 out]
                      }
                      n805 = call <vilib>:"Std Deviation and Variance.vi"("X"=w1769) -> ("mean"=w1768:dbl)  [unwired: 1 in, 2 out]
                      n806 = Divide(x=w1760, y=w1768) -> (x/y=w1766:dbl)
                      n807 = Reciprocal(x=w1766) -> (1/x=w1763:dbl)
                      n808 = Multiply(x=w1763, y=1000.0) -> (x*y=w1756:dbl)
                      n809 = Number To Fractional String(number=w1756, precision (6)=i16 2) -> (F-format string=w1752:string)  [unwired: 2 in]
                      n810 = Divide(x=w1763, y=9.81) -> (x/y=w1759:dbl)
                      n811 = In Range and Coerce(upper limit=14.5, x=w1756, lower limit=7.5) -> (In Range?=w1750:bool)  [unwired: 1 out]
                      n812 = Select(t="\n\nACCELEROMETER CALIBRATED CORRECTLY\n------------------------------------------------------------------------ \n", s=w1750, f="\n\nCALIBRATION FAILED\nSENSITIVITY OUT OF RANGE (7,5-14,5)\n------------------------------------------------------------------------ \n") -> (s? t:f=w1751:string)
                      n813 = Concatenate Strings("\nAMPLITUDE CALIBRATION:\n\nSENSIVITY: ", w1752, w1751, "\r") -> (w1749:string)
                    }
                  }
                  n814 = local read "Report"() -> (w1742:string)
                  n815 = Concatenate Strings(w1734, w1742) -> (w1741:string)
                  n816 = local write "Report"(w1741) -> ()
                  "Calibration parameter" <- w1739
                }
              }
              n817 = Wait Until Next ms Multiple(millisecond multiple=u32 200 ("milliseconds to wait")) -> ()  [unwired: 1 out]
              n818 = Not(x=w1033) -> (.not. x?=w1039:bool)
              n819 = Concatenate Strings(w1035, w1037) -> (w1036:string)
              "Numeric" <- w1034
            }
            n820 = while {
              tunnel: [w1010] -> w990
              tunnel: w991 -> [w1010]
              i -> [w1007]
              stop <- w1008 stop-if-true
              n821 = Wait (ms)(milliseconds to wait=u32 1000) -> ()  [unwired: 1 out]
              n822 = Greater?(x=w1007, y=2) -> (0:w1008:bool)
            }
            n823 = local read "calibration log"() -> (w997:path)
            n824 = Write to Text File(file (use dialog)=w997, text=w990) -> ()  [unwired: 2 in, 3 out]
            n825 = flat-sequence {
              tunnel: w996 -> [w1019]
              tunnel: w992 -> [w1018]
              tunnel: [w1019] -> w995
              tunnel: [w1018] -> w993
              frame #0 {
                # "Antes Accel. detected"
                n826 = local read "Accelerometer"() -> (w1016:i32)
                n827 = local read "Save calibration"() -> (w1015:bool)
                n828 = Add(x=w1016, y=7) -> (x+y=w1013:i32)
                n829 = Less Or Equal?(x=w1013, y=15) -> (x <= y?=w1014:bool)
                n830 = And(x=w1014, y=w1015) -> (x .and. y?=w1011:bool)
                n831 = case shown="True" w1011 {
                  tunnel: w1013 -> [_ w1020]
                  frame False {
                  }
                  frame True {
                    w1030 = "Parametros"  # Key 1
                    n832 = local read "configuration file path"() -> (w1022:path)
                    n833 = local read "Calibration parameter"() -> (w1021:dbl)
                    n834 = Number To Decimal String(number=w1020) -> (decimal integer string=w1031:string)  [unwired: 1 in]
                    n835 = Concatenate Strings(w1030, w1031) -> (w1024:string)
                    n836 = call <vilib>:"Open Config Data.vi"("create file if necessary (T)"=TRUE, "configuration file path"=w1022) -> ("error out"=w1025:errorcluster, "refnum"=w1026:T13)  [unwired: 1 in, 7 out]
                    n837 = call-poly <vilib>:"Write Key.vi"("section"="Adquisicion", "error in (no error)"=w1025, "value"=w1021, "key"=w1024, "refnum"=w1026) -> ("error out"=w1029:errorcluster, "refnum out"=w1028:T13)  [unwired: 3 in, 2 out]
                    n838 = call <vilib>:"Close Config Data.vi"("error in (no error)"=w1029, "refnum"=w1028) -> ()  [unwired: 8 in, 2 out]
                  }
                }
              }
            }
          }
          frame "UPS" {
            n839 = flat-sequence {
              tunnel: w1792 -> [w1804]
              tunnel: [w1804] -> w1791
              frame #0 {
                n840 = local read "Report"() -> (w1803:string)
                n841 = call "Reporting_datetime.vi"() -> ("String"=w1801:string)  [unwired: 11 in]
                n842 = Concatenate Strings(w1801, "\nSTATUS: UPS\n\n", w1803) -> (w1802:string)
                n843 = local write "Report"(w1802) -> ()
              }
            }
            n844 = node-c288() -> (w1799:T7)  [unwired: 4 in]
            n845 = timed-loop {
              timing: w1799 -> [_]
              timing-out: [_] -> w1798
              tunnel: w1797 -> [w1813]
              tunnel: w1791 -> [w1812]
              tunnel: [w1811] -> w1796
              tunnel: [w1810] -> w1795
              stop <- w1805 stop-if-true
              n846 = node-c288() -> ()  [unwired: 1 in, 1 out]
              n847 = xnode "Read/Write Control"("FPGA VI Reference In"=w1813, "error in"=w1812) -> ("FPGA VI Reference Out"=w1811:refnum<k20>, "error out"=w1810:errorcluster, "DC OK"=w1808:bool, "Chassis Temperature"=w1809:i16)
              n848 = call "ControlTemperatura.vi"("Chassis Temperature"=w1809) -> ("T fuera rango"=w1807:bool)  [unwired: 2 out]
              n849 = Not(x=w1807) -> (.not. x?=w1806:bool)
              n850 = And(x=w1808, y=w1806) -> (x .and. y?=w1805:bool)
              n851 = node-c288() -> ()  [unwired: 1 in, 1 out]
            }
            n852 = node-c288(w1798) -> ()  [unwired: 1 out]
          }
          frame "Diagnosis" {
            (unwired) "%Y/%m/%d %H:%M:%S" ("time format string (%c)")
            n853 = flat-sequence {
              tunnel: w1838 -> [w2050]
              tunnel: [w2050] -> w1837
              frame #0 {
                n854 = local read "Report"() -> (w2049:string)
                n855 = call "Reporting_datetime.vi"() -> ("String"=w2047:string)  [unwired: 11 in]
                n856 = Concatenate Strings(w2047, "\nSTATUS: AUTODIAGNOSIS\n\n", w2049) -> (w2048:string)
                n857 = local write "Report"(w2048) -> ()
              }
            }
            n858 = xnode "Invoke Method"("FPGA VI Reference In"=w1836, "error in"=w1837) -> ("FPGA VI Reference Out"=w1828:refnum<k20>, "error out"=w1829:errorcluster)  [unwired: 1 in]
            n859 = flat-sequence {
              tunnel: [w1865] -> w1835
              tunnel: [w1864] -> w1834
              tunnel: [w1855] -> w1833
              tunnel: [w1854] -> w1832
              tunnel: w1829 -> [w1843]
              tunnel: w1828 -> [w1844]
              tunnel: [w1847] -> w1824
              tunnel: [w1846] -> w1823
              tunnel: w1835 -> [w1889]
              tunnel: w1834 -> [w1890]
              tunnel: w1833 -> [w1887]
              tunnel: w1832 -> [w1886]
              tunnel: [w1888] -> w1831
              tunnel: [w1884] -> w1830
              tunnel: w1824 -> [w1879]
              tunnel: w1823 -> [w1878]
              tunnel: [w1875] -> w1822
              tunnel: w1831 -> [w1962]
              tunnel: w1830 -> [w1963]
              tunnel: w1822 -> [w1955]
              tunnel: [w1977] -> w1821
              tunnel: [w1976] -> w1820
              tunnel: [w2044] -> w1827
              tunnel: [w2045] -> w1818
              tunnel: w1821 -> [w2045]
              tunnel: w1820 -> [w2044]
              frame #0 {
                w1845 = sgl[] [] ("A1")
                n860 = local read "Frecuencia de muestreo y módulo CRIO"() -> (w1863:T3)
                n861 = xnode "Read/Write Control"("FPGA VI Reference In"=w1844, "error in"=w1843) -> ("FPGA VI Reference Out"=w1842:refnum<k20>, "error out"=w1841:errorcluster, "DC OK"=→"Power Status":bool)
                n862 = local read "Escaneos de la FIFO por canal"() -> (w1860:u32)
                n863 = local read "Frecuencia de muestreo (Hz)"() -> (w1861:dbl)
                n864 = local read "Nº de acelerómetros"() -> (w1858:i32)
                n865 = Get Date/Time In Seconds() -> (seconds since 1Jan1904=→"Inicio diagnosis":timestamp)
                n866 = local read "Nº inductivos"() -> (w1859:i32)
                n867 = local read "Canal cero WS2"() -> (w1852:bool)
                n868 = local read "Canal cero WS1?"() -> (w1853:bool)
                n869 = local read "Count(mSec)"() -> (w1862:u32)
                n870 = xnode "Read/Write Control"("FPGA VI Reference In"=w1842, "error in"=w1841, "Fotocélula"=TRUE ("Adquirir")) -> ("FPGA VI Reference Out"=w1869:refnum<k20>, "error out"=w1868:errorcluster)
                n871 = Add(x=w1859, y=w1858) -> (x+y=w1857:i32)
                n872 = call "DMACalc.vi"("Number of Channels"=w1857, "Number of Samples"=w1860, "Rate (Hz)"=w1861) -> ("Block Size"=w1854:u32, "Time to Acquire Block (ms)"=w1855:i32, "Host Buffer Size"=w1856:u32)  [unwired: 6 in]
                n873 = xnode "Read/Write Control"("FPGA VI Reference In"=w1869, "error in"=w1868, "Data Rate"=w1863, "Digital?"=FALSE, "Count(mSec)"=w1862, "Canal cero WS1?"=w1853, "Canal cero WS2?"=w1852) -> ("FPGA VI Reference Out"=w1871:refnum<k20>, "error out"=w1870:errorcluster)
                n874 = xnode "Invoke Method"("FPGA VI Reference In"=w1871, "error in"=w1870, "Requested Depth"=w1856) -> ("FPGA VI Reference Out"=w1873:refnum<k20>, "error out"=w1872:errorcluster)  [unwired: 1 out]
                n875 = Open/Create/Replace File(file path (use dialog)=path "c:/diagnosis.bin" ("file (use dialog)"), operation (0:open)=T5."replace or create", access (0:read/write)=enum16{"read/write", "read-only", "write-only"}."read/write", disable buffering (F)=TRUE) -> (refnum out=w1847:refnum<file>, error out=w1846:errorcluster)  [unwired: 1 in, 2 out]
                n876 = xnode "Invoke Method"("FPGA VI Reference In"=w1873, "error in"=w1872) -> ("FPGA VI Reference Out"=w1865:refnum<k20>, "error out"=w1864:errorcluster)
                n877 = local write "A1"(w1845) -> ()
                n878 = local write "A2"(w1845) -> ()
                n879 = local write "A3"(w1845) -> ()
                n880 = local write "A4"(w1845) -> ()
                n881 = local write "A5"(w1845) -> ()
                n882 = local write "A6"(w1845) -> ()
                n883 = local write "A7"(w1845) -> ()
                n884 = local write "A8"(w1845) -> ()
                n885 = local write "I1"(w1845) -> ()
                n886 = local write "I2"(w1845) -> ()
              }
              frame #1 {
                n887 = while "Data Acquisition" {
                  tunnel: w1889 -> [w1918]
                  shift-right: [w1922] -> _
                  shift-left: u32 0 ("t") -> [w1897]
                  tunnel: w1887 -> [w1923]
                  tunnel: w1886 -> [w1921]
                  shift-right: [w1924] -> w1884
                  shift-left: w1890 -> [w1917]
                  tunnel: [w1919] -> w1888
                  tunnel: w1879 -> [w1895]
                  shift-right: [w1892] -> w1877
                  shift-left: w1878 -> [w1894]
                  tunnel: [w1893] -> w1876
                  stop <- w1920 stop-if-true
                  # "Detector de presencia"
                  # "Mide el tiempo de paso del tren y con ello se puede calcular\nla velocidad la unidad"
                  n888 = xnode "Invoke Method"("FPGA VI Reference In"=w1918, "error in"=w1917, "Number of Elements"=w1897, "Timeout (ms)"=0) -> ("FPGA VI Reference Out"=w1910:refnum<k20>, "error out"=w1909:errorcluster, "Data"=w1916:fxp<+/-,24,4>[], "Elements Remaining"=w1898:u32)
                  n889 = case "Data Ready" shown="Default" w1897 {
                    tunnel: w1923 -> [w1929 _]
                    tunnel: [w1927 u32 0 ("t")] -> w1922
                    tunnel: w1921 -> [w1930 _]
                    tunnel: w1898 -> [w1928 _]
                    tunnel: w1916 -> [_ w1944]
                    tunnel: w1894 -> [w1926 w1941]
                    tunnel: [w1926 w1939] -> w1892
                    tunnel: w1895 -> [w1925 w1938]
                    tunnel: [w1925 w1937] -> w1893
                    frame 0 {
                      n890 = Greater Or Equal?(x=w1928, y=w1930) -> (x >= y?=w1931:bool)
                      n891 = case shown="False" w1931 {
                        tunnel: [u32 0 ("Block Size") w1935] -> w1927
                        tunnel: [w1934 0 ("t")] -> w1932
                        tunnel: w1929 -> [w1934 _]
                        tunnel: w1930 -> [_ w1935]
                        frame False {
                        }
                        frame True {
                        }
                      }
                      n892 = call "WaitMinTimeBetweenCall.vi"("Minimum ms between calls"=w1932) -> ()  [unwired: 2 in]
                    }
                    frame Default {
                      n893 = To Single Precision Float(number=w1944) -> (single precision float=w1940:sgl[])
                      n894 = Write to Binary File(file (use dialog)=w1938, data=w1940, error in=w1941, 5:FALSE ("prepend array or string size? (T)"), 9:T6."little-endian" ("byte order (0:big-endian, network order)")) -> (refnum out=w1937:refnum<file>, error out=w1939:errorcluster)  [unwired: 2 out]
                    }
                  }
                  n895 = xnode ("CheckLate")("FPGA VI Reference In"=w1910, "error in"=w1909) -> ("FPGA VI Reference Out"=w1905:refnum<k20>, "error out"=w1914:errorcluster, "Buffer Underflow"=w1900:bool, "Buffer Overflow"=w1901:bool)
                  n896 = local read "Inicio diagnosis"() -> (w1902:timestamp)
                  n897 = Get Date/Time In Seconds() -> (seconds since 1Jan1904=w1903:timestamp)
                  n898 = To Double Precision Float(number=w1902) -> (double precision float=w1908:dbl)
                  n899 = To Double Precision Float(number=w1903) -> (double precision float=w1907:dbl)
                  n900 = local write "Buffer Overflow"(w1901) -> ()
                  n901 = Subtract(x=w1907, y=w1908) -> (x-y=w1911:dbl)
                  n902 = local write "Buffer Underflow"(w1900) -> ()
                  n903 = Greater?(x=w1911, y=1.0 ("Tiempo de adquisición")) -> (0:w1906:bool)
                  n904 = call "ErrorOverFlow.vi"("Buffer Overflow"=w1901) -> ("error out"=w1912:errorcluster)
                  n905 = call "ErrorUnderFlow.vi"("Buffer Overflow"=w1900) -> ("error out"=w1913:errorcluster)
                  n906 = Unbundle By Name(w1892) -> ("status"=w1891:bool)
                  n907 = Merge Errors(w1914, w1913, w1912) -> (w1896:errorcluster)
                  n908 = Unbundle By Name(w1896) -> ("status"=w1915:bool)
                  n909 = Compound Arithmetic op=OR(w1915, w1906, w1891) -> (w1920:bool)
                  n910 = case "Flush" shown="True" w1920 {
                    tunnel: w1905 -> [w1946 w1951]
                    tunnel: w1896 -> [w1947 w1950]
                    tunnel: [w1947 w1949] -> w1924
                    tunnel: [w1946 w1948] -> w1919
                    frame False {
                    }
                    frame True {
                      n911 = xnode "Invoke Method"("FPGA VI Reference In"=w1951, "error in"=w1950) -> ("FPGA VI Reference Out"=w1948:refnum<k20>, "error out"=w1949:errorcluster)
                    }
                  }
                }
                n912 = local read "Report"() -> (w1883:string)
                n913 = call "Reporting_error.vi"("error out 2"=w1884, "Concept"="FPGA ") -> ("Reporting"=w1885:string)  [unwired: 1 in]
                n914 = Close File(refnum=w1876, error in=w1877) -> (path=w1875:path)  [unwired: 1 out]
                n915 = Concatenate Strings(w1885, w1883) -> (w1880:string)
                n916 = local write "Report"(w1880) -> ()
              }
              frame #2 {
                n917 = xnode "Read/Write Control"("FPGA VI Reference In"=w1962, "error in"=w1963) -> ("FPGA VI Reference Out"=w1960:refnum<k20>, "error out"=w1961:errorcluster, "Direccion 0?"=w1959:bool)
                n918 = Read from Binary File(5:sgl 1.25, 9:T6."little-endian" ("byte order (0:big-endian, network order)"), 10:-1 ("count (1)"), 11:w1955) -> (0:w1953:errorcluster, 2:w1954:sgl[], 3:w1952:refnum<file>)  [unwired: 1 in, 2 out]
                "Diagnostic data" <- w1954
                n919 = local write "Direccion 0?"(w1959) -> ()
                n920 = Close File(refnum=w1952, error in=w1953) -> ()  [unwired: 2 out]
                n921 = Decimate 1D Array(w1954) -> (w1968:sgl[], w1965:sgl[], w1966:sgl[], w1967:sgl[], w1969:sgl[], w1970:sgl[], w1971:sgl[], w1972:sgl[], w1973:sgl[], w1974:sgl[])
                n922 = Build Array(w1968, w1965, w1966, w1967, w1969, w1970, w1971, w1972, w1973, w1974) -> (w1964:sgl[][])
                n923 = xnode "Read/Write Control"("FPGA VI Reference In"=w1960, "error in"=w1961, "Stop"=TRUE) -> ("FPGA VI Reference Out"=w1978:refnum<k20>, "error out"=w1979:errorcluster)
                n924 = for {
                  tunnel: w1964 -> [w1980] mode=indexing
                  i -> [w1981]
                  n925 = case shown="9" w1981 {
                    tunnel: w1980 -> [w1982 w1983 w1984 w1985 w1986 w1987 w1988 w1989 w1990 w1991 _]
                    frame 0 {
                      "A1" <- w1982
                    }
                    frame 1 {
                      "A2" <- w1983
                    }
                    frame 2 {
                      "A3" <- w1984
                    }
                    frame 3 {
                      "A4" <- w1985
                    }
                    frame 4 {
                      "A5" <- w1986
                    }
                    frame 5 {
                      "A6" <- w1987
                    }
                    frame 6 {
                      "A7" <- w1988
                    }
                    frame 7 {
                      "A8" <- w1989
                    }
                    frame 8 {
                      "I1" <- w1990
                    }
                    frame 9 {
                      "I2" <- w1991
                    }
                    frame 10, Default {
                    }
                  }
                }
                n926 = xnode "Invoke Method"("FPGA VI Reference In"=w1978, "error in"=w1979) -> ("FPGA VI Reference Out"=w1977:refnum<k20>, "error out"=w1976:errorcluster)
              }
              frame #3 {
                n927 = local read "Puerto RFID"() -> (w2038:u16)
                n928 = local read "configuration file path"() -> (w2031:path)
                n929 = local read "IP RFID"() -> (w2039:string)
                n930 = local read "RFID_status"() -> (w2041:path)
                n931 = call "Read_diagnosis_data.vi"("configuration file path"=w2031) -> ("acelerometros"=w2022:dbl, "WD"=w2035:dbl)  [unwired: 9 in]
                n932 = call "conexion_internet.vi"() -> ("Internet status"=w2005:string, "Internet connection"=→"Internet connection":bool)  [unwired: 10 in]
                n933 = call "RFID_connection.vi"("Puerto RFID"=w2038, "IP RFID"=w2039) -> ("RFID_connection_text"=w2004:string, "RFID connection"=→"RFID connection":bool)  [unwired: 8 in]
                n934 = call "show_tag_status.vi"("file path (dialog if empty)"=w2041) -> ("Output"=→"Last Train passes - RFIDs":T1, "train_passes_text"=w2003:string)  [unwired: 9 in]
                n935 = local read "Direccion 0?"() -> (w2034:bool)
                n936 = local read "I1"() -> (w2033:sgl[])
                n937 = local read "I2"() -> (w2032:sgl[])
                n938 = local read "A1"() -> (w2021:sgl[])
                n939 = local read "A2"() -> (w2020:sgl[])
                n940 = local read "A3"() -> (w2014:sgl[])
                n941 = local read "A4"() -> (w2015:sgl[])
                n942 = local read "A5"() -> (w2016:sgl[])
                n943 = local read "A6"() -> (w2017:sgl[])
                n944 = local read "A7"() -> (w2018:sgl[])
                n945 = local read "A8"() -> (w2019:sgl[])
                n946 = call "Wheel_detector_status.vi"("WD_offset"=w2035, "I2"=w2032, "I1"=w2033, "Direccion 0?"=w2034) -> ("WD_status"=w2002:string, "I2"=→"Wheel detector 2":bool, "I1"=→"Wheel Detector 1":bool)  [unwired: 5 in]
                n947 = call "Accelerometer_status.vi"("Number"=1, "Acc_offset"=w2022, "Accelerometer"=w2021) -> ("Accelerometer_status"=w2001:string, "Accelerometer"=→"Accelerometer 1":bool)  [unwired: 7 in]
                n948 = call "Accelerometer_status.vi"("Number"=2, "Acc_offset"=w2022, "Accelerometer"=w2020) -> ("Accelerometer_status"=w2000:string, "Accelerometer"=→"Accelerometer 2":bool)  [unwired: 7 in]
                n949 = call "Accelerometer_status.vi"("Number"=3, "Acc_offset"=w2022, "Accelerometer"=w2014) -> ("Accelerometer_status"=w1999:string, "Accelerometer"=→"Accelerometer 3":bool)  [unwired: 7 in]
                n950 = call "Accelerometer_status.vi"("Number"=4, "Acc_offset"=w2022, "Accelerometer"=w2015) -> ("Accelerometer_status"=w1998:string, "Accelerometer"=→"Accelerometer 4":bool)  [unwired: 7 in]
                n951 = call "Accelerometer_status.vi"("Number"=5, "Acc_offset"=w2022, "Accelerometer"=w2016) -> ("Accelerometer_status"=w1997:string, "Accelerometer"=→"Accelerometer 5":bool)  [unwired: 7 in]
                n952 = call "Accelerometer_status.vi"("Number"=6, "Acc_offset"=w2022, "Accelerometer"=w2017) -> ("Accelerometer_status"=w1996:string, "Accelerometer"=→"Accelerometer 6":bool)  [unwired: 7 in]
                n953 = call "Accelerometer_status.vi"("Number"=7, "Acc_offset"=w2022, "Accelerometer"=w2018) -> ("Accelerometer_status"=w1995:string, "Accelerometer"=→"Accelerometer 7":bool)  [unwired: 7 in]
                n954 = call "Accelerometer_status.vi"("Number"=8, "Acc_offset"=w2022, "Accelerometer"=w2019) -> ("Accelerometer_status"=w1994:string, "Accelerometer"=→"Accelerometer 8":bool)  [unwired: 7 in]
                n955 = local read "Report"() -> (w1993:string)
                n956 = Concatenate Strings(w2005, w2004, w2003, w2002, w2001, w2000, w1999, w1998, w1997, w1996, w1995, w1994, w1993) -> (w1992:string)
                n957 = property on="Report" class="Str"("Value"=w1992) -> ()  [unwired: 2 in, 2 out]
              }
            }
            n958 = Get Date/Time In Seconds() -> (seconds since 1Jan1904=w1826:timestamp)
            n959 = Format Date/Time String(seconds (now)=w1826) -> (date/time string=→"Last time checked":string)  [unwired: 2 in]
          }
        }
        "error manipulacion archivos" <- w111
        n960 = local read "Parar la aplicación"() -> (w109:bool)
      }
      n961 = case shown="True" w82 {
        frame False {
        }
        frame True {
          w90 = T14 {"IP"="169.254.1.1", "Port"=5084, "ReaderConfigFile"=path "", "ROspecConfigFile"=path ""}  # RFID Configuration
          w94 = path "" ("ReaderConfigFile")
          # "Loop RFID reader"
          n962 = local read "Puerto RFID"() -> (w92:u16)
          n963 = local read "IP RFID"() -> (w93:string)
          n964 = Bundle By Name(cluster=w90, "IP"=w93, "Port"=w92, "ReaderConfigFile"=w94, "ROspecConfigFile"=w94) -> (w91:T14)
          n965 = while {
            tunnel: w91 -> [w96]
            stop <- w97 stop-if-true
            n966 = local read "Parar la aplicación"() -> (w97:bool)
            n967 = call "IF2_Reader.vi"("Stop"=w97, "RFID Configuration"=w96) -> ("error out"=w98:errorcluster, "connection ID"=→"connection ID":refnum<k5>)  [unwired: 8 in]
            n968 = case shown="Error" w98 {
              tunnel: w98 -> [_ w100]
              tunnel: [TRUE ("RFIDStatus") FALSE ("RFIDStatus")] -> _
              frame No Error {
              }
              frame Error {
                n969 = call "Reporting_error.vi"("error out 2"=w100, "Concept"="Passive RFID") -> ("Reporting"=w102:string)  [unwired: 1 in]
                n970 = local read "Report"() -> (w103:string)
                n971 = Concatenate Strings(w102, w103) -> (w101:string)
                n972 = local write "Report"(w101) -> ()
              }
            }
          }
        }
      }
      n973 = xnode "Close FPGA VI Reference"("FPGA VI Reference In"=w85, "error in"=w84) -> ("error out"=→"error FPGA":errorcluster)
    }
    frame #3 {
      n974 = call "LH6HD.vi"("Action"=enum16{"Init", "Start", "Read", "Stop", "Exit"}."Stop") -> ("error out"=→"RFID_LR6_Error":errorcluster)  [unwired: 9 in, 1 out]
    }
  }
